vi "Autonomous Independent.vi"   [LabVIEW 2016]
doc: "This VI is called when autonomous begins, and will automatically be terminated when autonomous ends. You can carry out timed or sensor driven robot movement independently without needing to return to the caller."
uses:
  <vilib>/Rock Robotics/Network Tables/NT Read String.vi
  Robot Global Data.vi
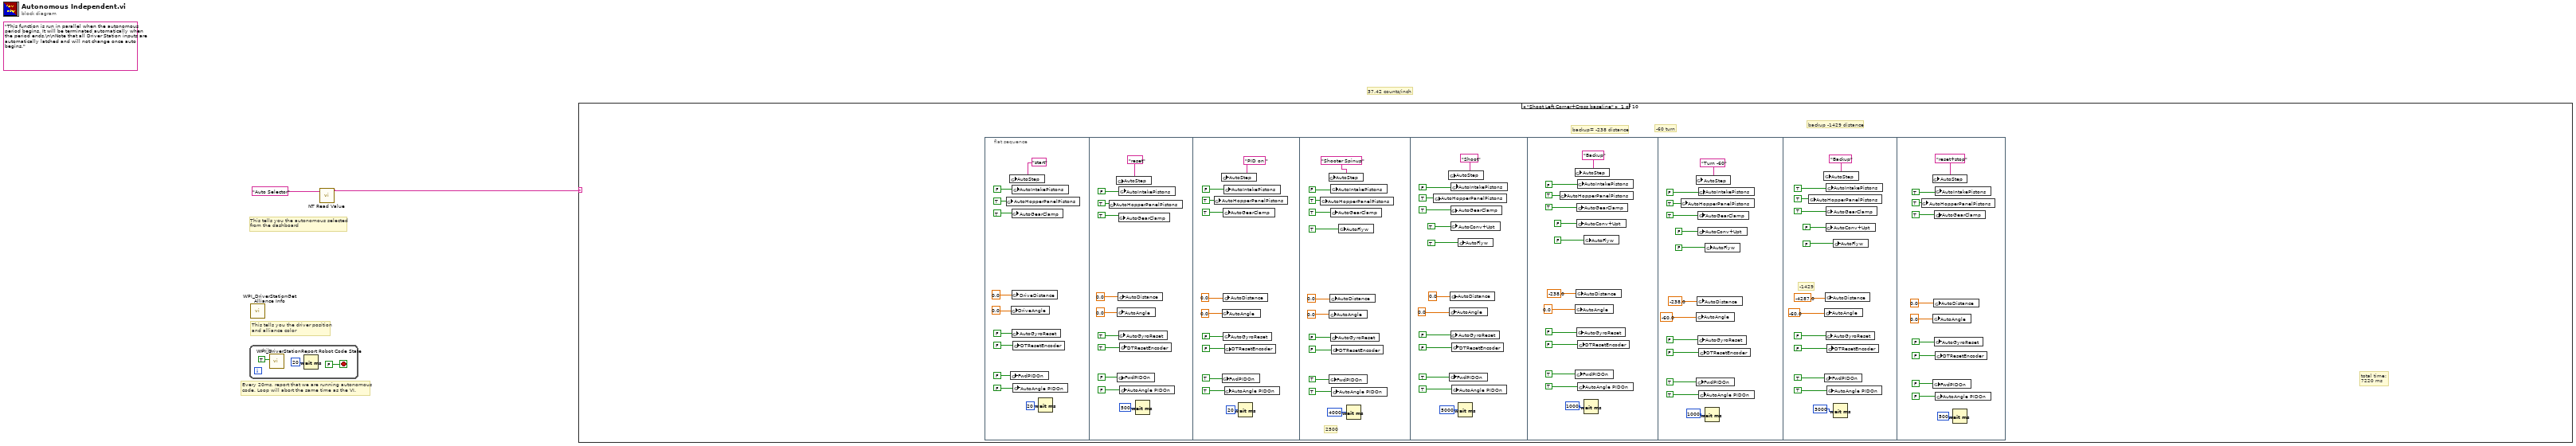
[diagram p0: block diagram]
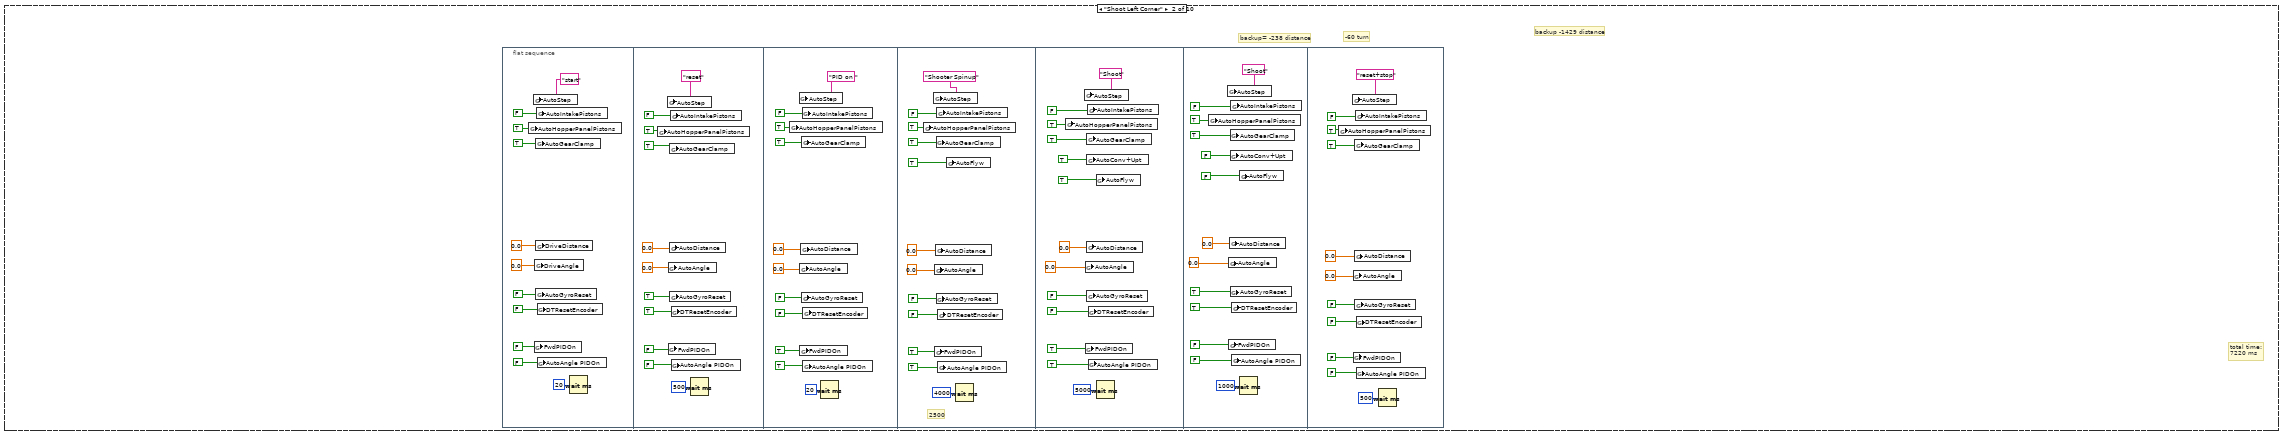
[diagram p2: hidden frame]
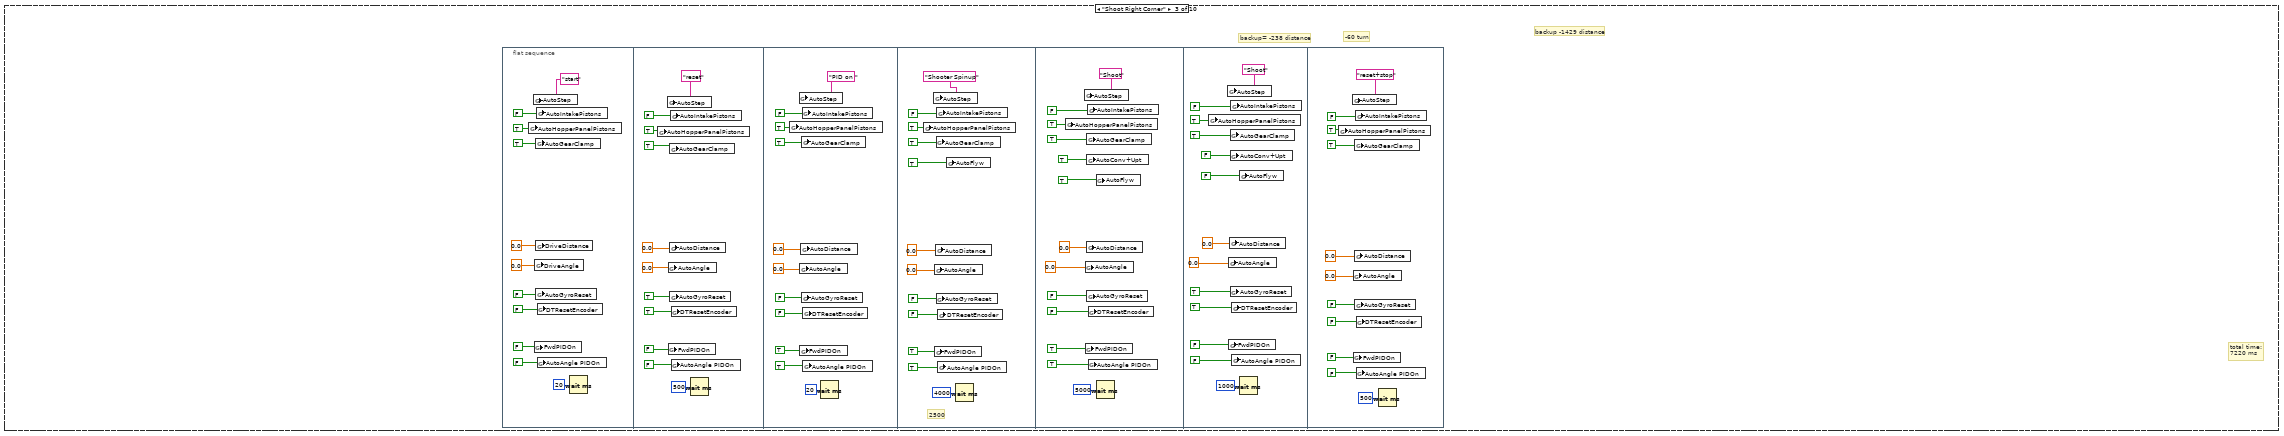
[diagram p3: hidden frame]
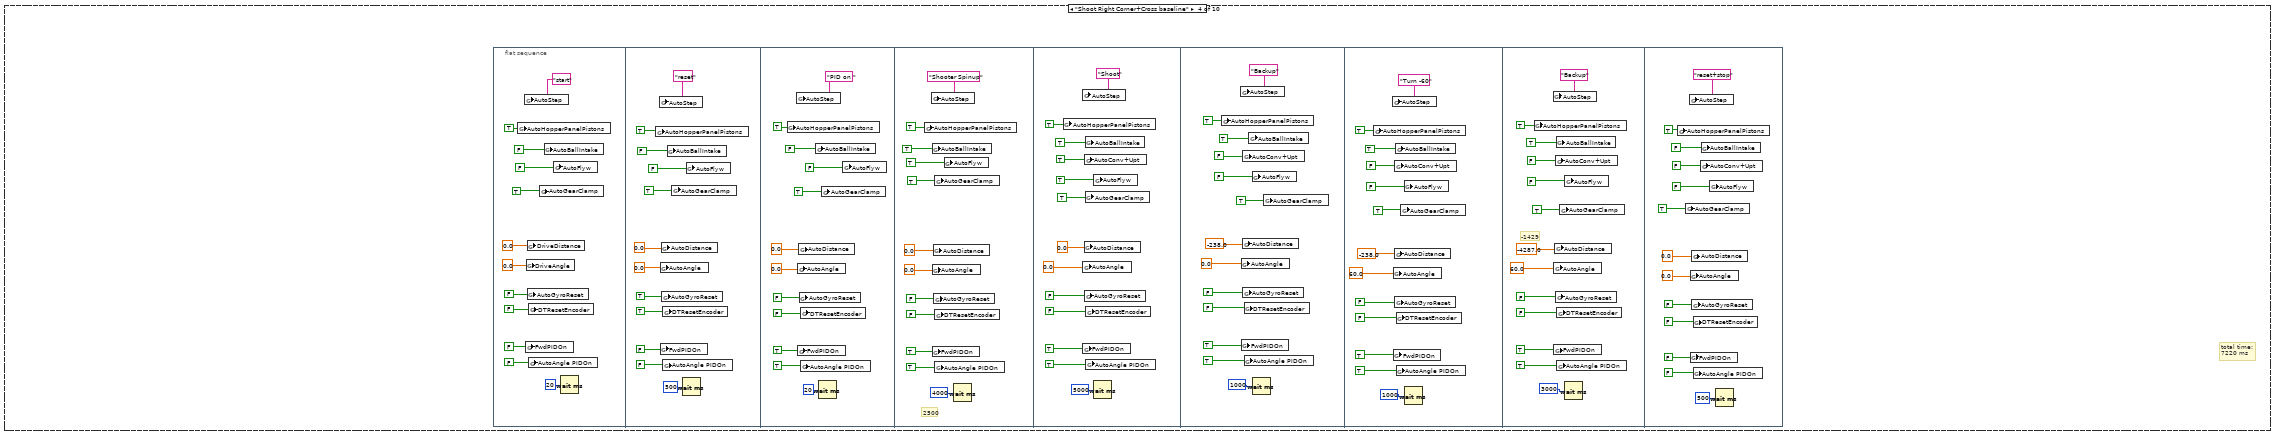
[diagram p4: hidden frame]
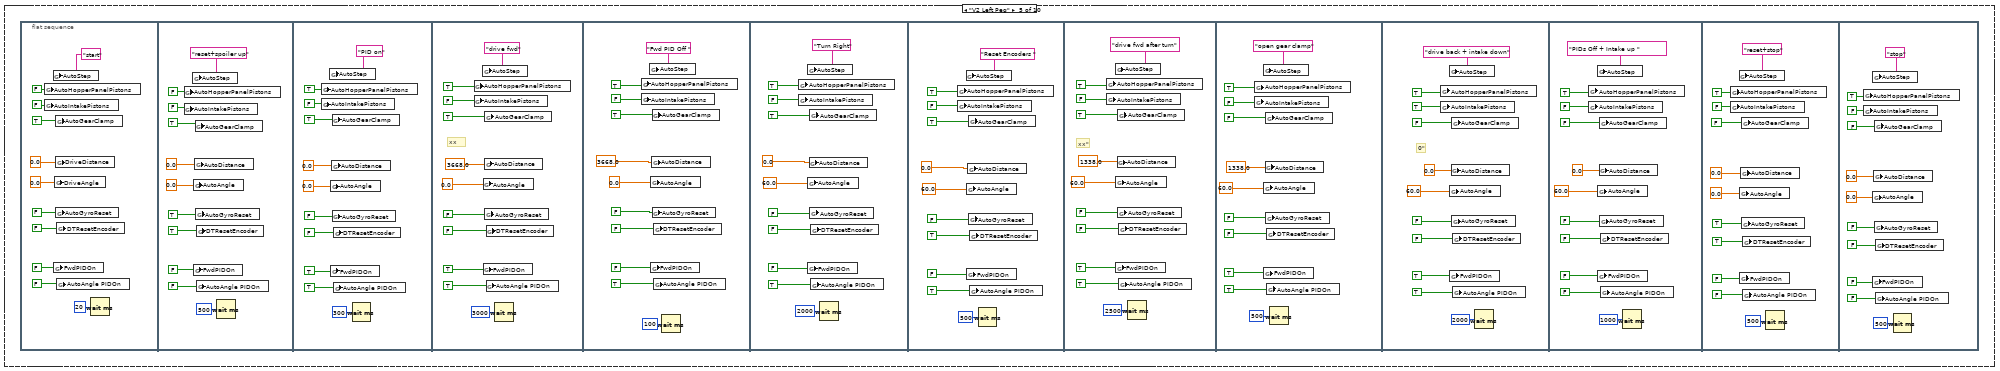
[diagram p5: hidden frame]
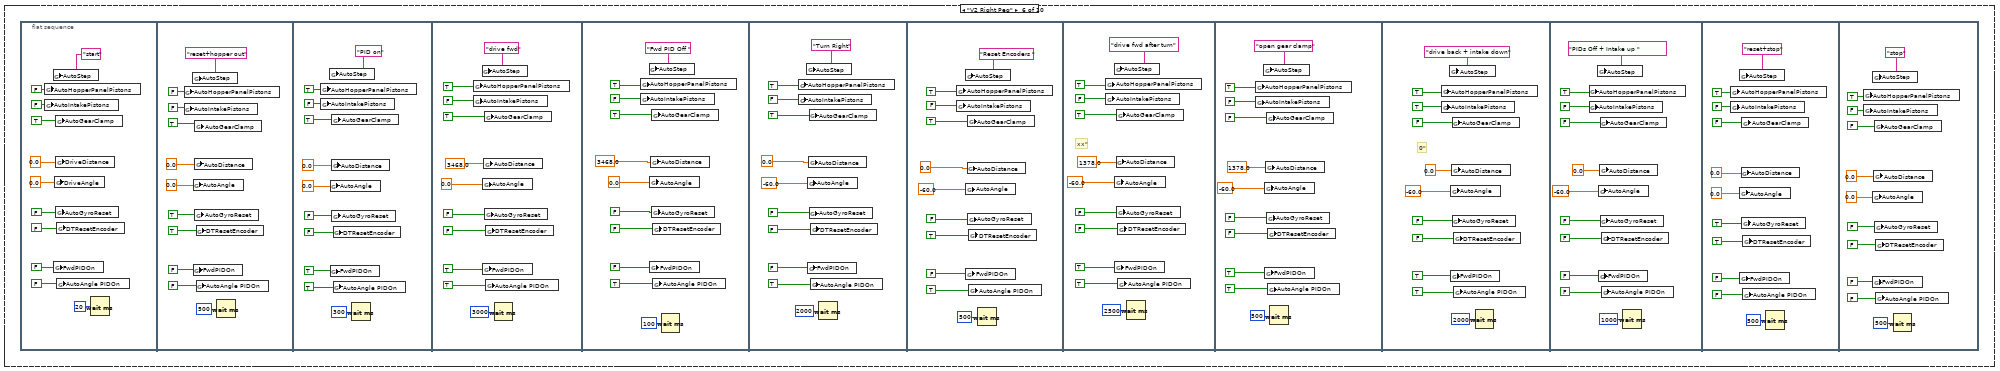
[diagram p6: hidden frame]
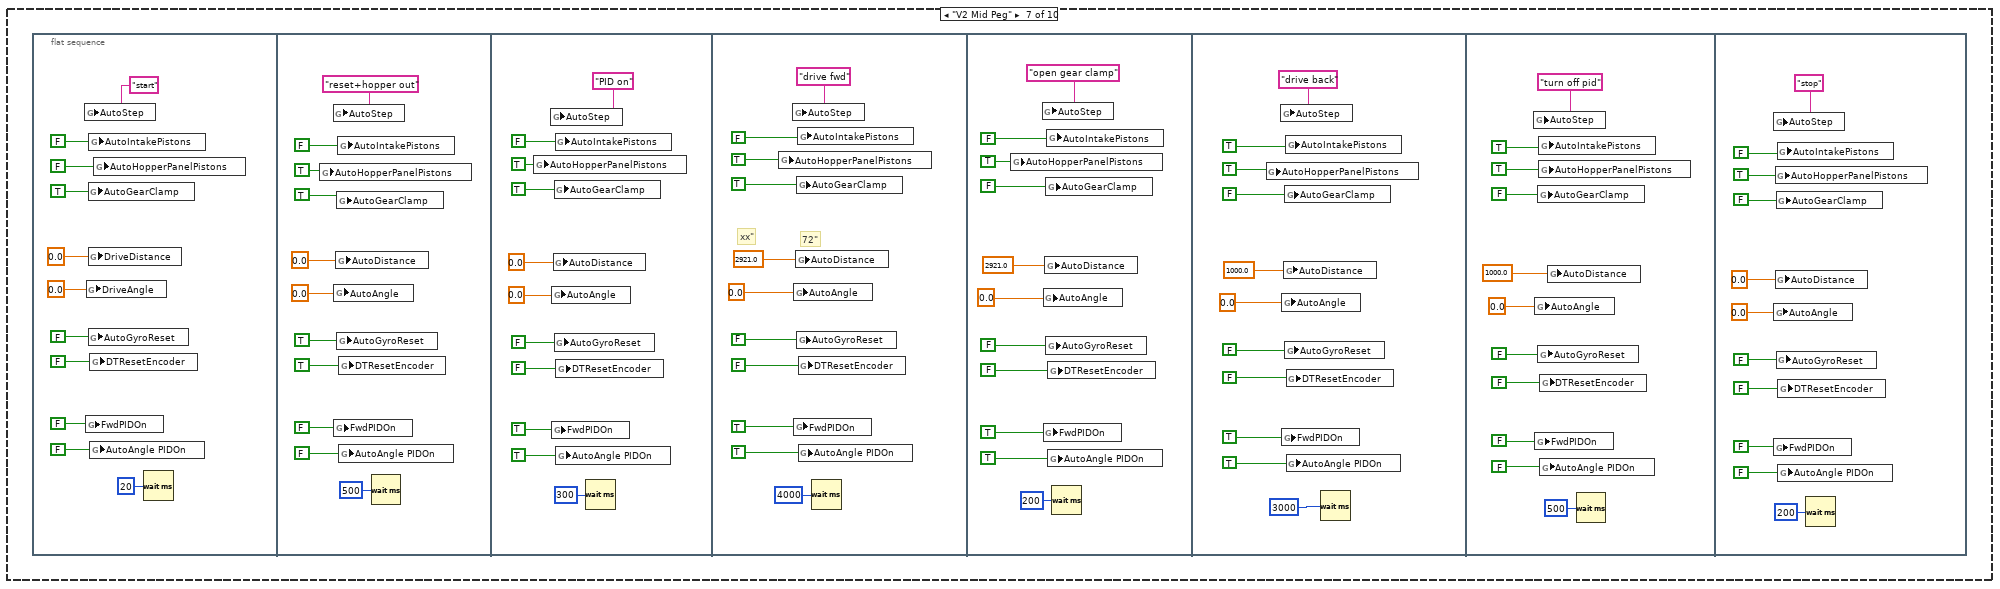
[diagram p7: hidden frame]
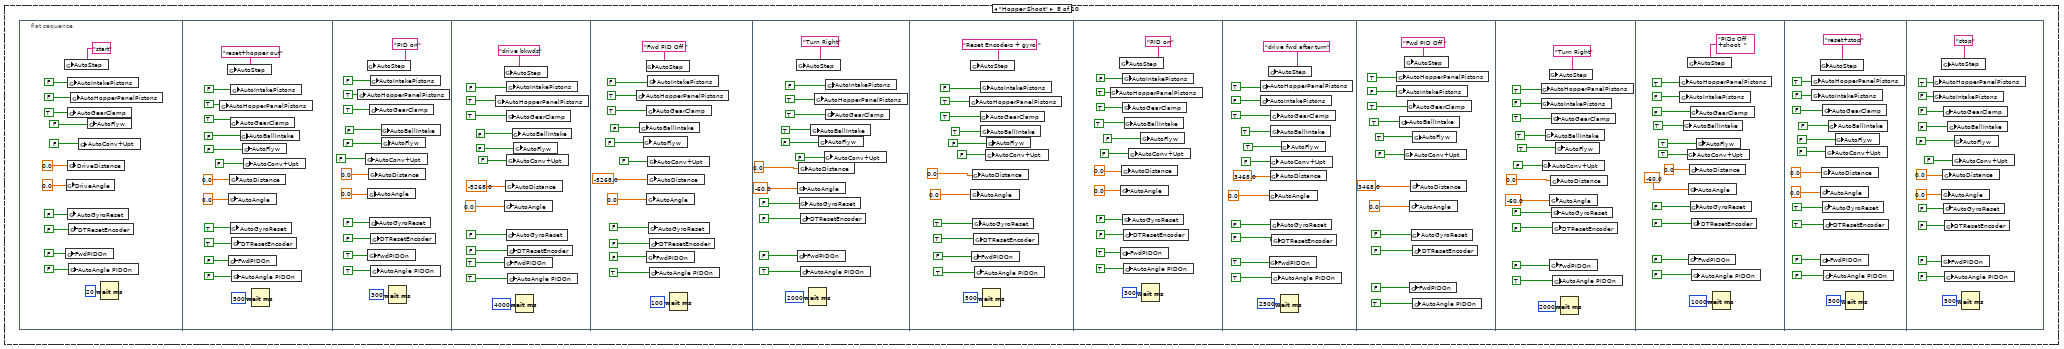
[diagram p8: hidden frame]
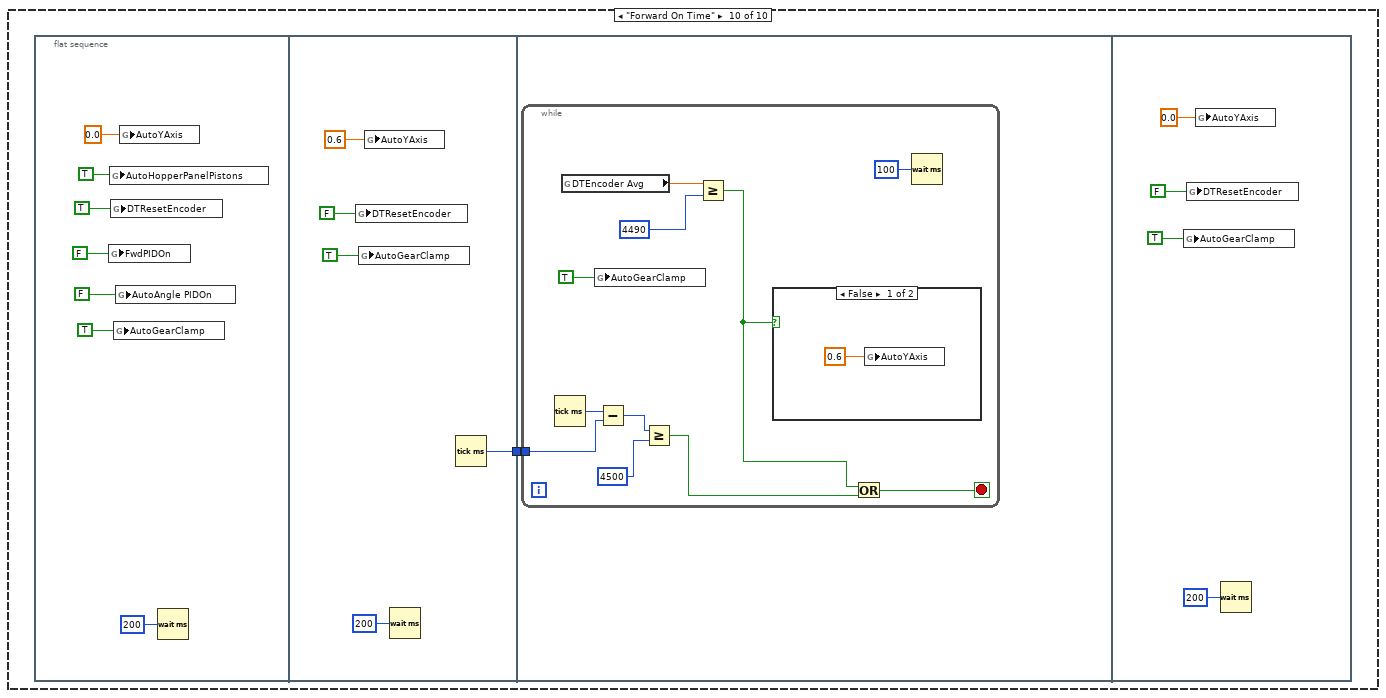
[diagram p10: hidden frame]
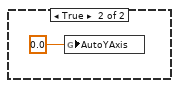
[diagram p11: hidden frame]
diagram:
  (unwired) "This function is run in parallel when the autonomous period begins. It will be terminated automatically when the period ends.\n\nNote that all Driver Station inputs are automatically latched and will not change once auto begins."
  # "37.42 counts/inch"
  # "This tells you the autonomous selected\nfrom the dashboard"
  # "Every 20ms, report that we are running autonomous\ncode. Loop will abort the same time as the VI."
  # "This tells you the driver position\nand alliance color"
  n1 = while {
    stop <- FALSE stop-if-true
    n2 = call <vilib>:"WPI_DriverStationReport Robot Code State.vi"("Autonomous"=TRUE) -> ()  [unwired: 10 in, 1 out]
    n3 = Wait (ms)(milliseconds to wait=u32 20) -> ()  [unwired: 1 out]
  }
  n4 = call <vilib>:"WPI_DriverStationGet Alliance Info.vi"() -> ()  [unwired: 12 out]
  n5 = call-poly <vilib>:"NT Read Value.vi"("Name"="Auto Selector") -> ("String"=w1:string)  [unwired: 9 in, 1 out]
  n6 = case shown="\"Shoot Left Corner+Cross baseline\"" w1 {
    frame "Shoot Left Corner+Cross baseline" {
      # "backup -1429 distance"
      # "-60 turn"
      # "backup= -238 distance"
      # "total time: \n7220 ms"
      n7 = flat-sequence {
        frame #0 {
          n8 = global write "Robot Global Data.vi" "AutoHopperPanelPistons"(TRUE ("GyroReset")) -> ()
          n9 = global write "Robot Global Data.vi" "AutoStep"("start" ("AutoStep")) -> ()
          n10 = global write "Robot Global Data.vi" "FwdPIDOn"(FALSE ("FwdPIDOn")) -> ()
          n11 = global write "Robot Global Data.vi" "DriveAngle"(0.0 ("DriveAngle")) -> ()
          n12 = global write "Robot Global Data.vi" "AutoGearClamp"(TRUE ("DTResetEncoder")) -> ()
          n13 = global write "Robot Global Data.vi" "DriveDistance"(0.0 ("DriveDistance")) -> ()
          n14 = global write "Robot Global Data.vi" "AutoGyroReset"(FALSE ("GyroReset")) -> ()
          n15 = global write "Robot Global Data.vi" "AutoIntakePistons"(FALSE ("GyroReset")) -> ()
          n16 = global write "Robot Global Data.vi" "DTResetEncoder"(FALSE ("DTResetEncoder")) -> ()
          n17 = global write "Robot Global Data.vi" "AutoAngle PIDOn"(FALSE ("AnglePIDOn")) -> ()
          n18 = Wait (ms)(milliseconds to wait=u32 20) -> ()  [unwired: 1 out]
        }
        frame #1 {
          n19 = global write "Robot Global Data.vi" "AutoHopperPanelPistons"(TRUE ("GyroReset")) -> ()
          n20 = global write "Robot Global Data.vi" "AutoStep"("reset" ("AutoStep")) -> ()
          n21 = global write "Robot Global Data.vi" "AutoAngle"(0.0 ("DriveAngle")) -> ()
          n22 = global write "Robot Global Data.vi" "FwdPIDOn"(FALSE ("FwdPIDOn")) -> ()
          n23 = global write "Robot Global Data.vi" "AutoDistance"(0.0 ("DriveDistance")) -> ()
          n24 = global write "Robot Global Data.vi" "AutoGearClamp"(TRUE ("DTResetEncoder")) -> ()
          n25 = global write "Robot Global Data.vi" "AutoGyroReset"(TRUE ("GyroReset")) -> ()
          n26 = global write "Robot Global Data.vi" "AutoIntakePistons"(FALSE ("GyroReset")) -> ()
          n27 = global write "Robot Global Data.vi" "DTResetEncoder"(TRUE ("DTResetEncoder")) -> ()
          n28 = global write "Robot Global Data.vi" "AutoAngle PIDOn"(FALSE ("AnglePIDOn")) -> ()
          n29 = Wait (ms)(milliseconds to wait=u32 500) -> ()  [unwired: 1 out]
        }
        frame #2 {
          n30 = global write "Robot Global Data.vi" "AutoHopperPanelPistons"(TRUE ("GyroReset")) -> ()
          n31 = global write "Robot Global Data.vi" "AutoStep"("PID on " ("AutoStep")) -> ()
          n32 = global write "Robot Global Data.vi" "AutoAngle"(0.0 ("DriveAngle")) -> ()
          n33 = global write "Robot Global Data.vi" "FwdPIDOn"(TRUE ("FwdPIDOn")) -> ()
          n34 = global write "Robot Global Data.vi" "AutoDistance"(0.0 ("DriveDistance")) -> ()
          n35 = global write "Robot Global Data.vi" "AutoGearClamp"(TRUE ("DTResetEncoder")) -> ()
          n36 = global write "Robot Global Data.vi" "AutoGyroReset"(FALSE ("GyroReset")) -> ()
          n37 = global write "Robot Global Data.vi" "AutoIntakePistons"(FALSE ("GyroReset")) -> ()
          n38 = global write "Robot Global Data.vi" "DTResetEncoder"(FALSE ("DTResetEncoder")) -> ()
          n39 = global write "Robot Global Data.vi" "AutoAngle PIDOn"(TRUE ("AnglePIDOn")) -> ()
          n40 = Wait (ms)(milliseconds to wait=u32 20) -> ()  [unwired: 1 out]
        }
        frame #3 {
          # "2500"
          n41 = global write "Robot Global Data.vi" "AutoHopperPanelPistons"(TRUE ("GyroReset")) -> ()
          n42 = global write "Robot Global Data.vi" "AutoStep"("Shooter Spinup" ("AutoStep")) -> ()
          n43 = global write "Robot Global Data.vi" "AutoAngle"(0.0 ("DriveAngle")) -> ()
          n44 = global write "Robot Global Data.vi" "FwdPIDOn"(TRUE ("FwdPIDOn")) -> ()
          n45 = global write "Robot Global Data.vi" "AutoDistance"(0.0 ("DriveDistance")) -> ()
          n46 = global write "Robot Global Data.vi" "AutoGearClamp"(TRUE ("DTResetEncoder")) -> ()
          n47 = global write "Robot Global Data.vi" "AutoGyroReset"(FALSE ("GyroReset")) -> ()
          n48 = global write "Robot Global Data.vi" "AutoIntakePistons"(FALSE ("GyroReset")) -> ()
          n49 = global write "Robot Global Data.vi" "DTResetEncoder"(FALSE ("DTResetEncoder")) -> ()
          n50 = global write "Robot Global Data.vi" "AutoAngle PIDOn"(TRUE ("AnglePIDOn")) -> ()
          n51 = global write "Robot Global Data.vi" "AutoFlyw"(TRUE ("DTResetEncoder")) -> ()
          n52 = Wait (ms)(milliseconds to wait=u32 4000) -> ()  [unwired: 1 out]
        }
        frame #4 {
          n53 = global write "Robot Global Data.vi" "AutoHopperPanelPistons"(TRUE ("GyroReset")) -> ()
          n54 = global write "Robot Global Data.vi" "AutoStep"("Shoot" ("AutoStep")) -> ()
          n55 = global write "Robot Global Data.vi" "AutoAngle"(0.0 ("DriveAngle")) -> ()
          n56 = global write "Robot Global Data.vi" "FwdPIDOn"(TRUE ("FwdPIDOn")) -> ()
          n57 = global write "Robot Global Data.vi" "AutoDistance"(0.0 ("DriveDistance")) -> ()
          n58 = global write "Robot Global Data.vi" "AutoGearClamp"(TRUE ("DTResetEncoder")) -> ()
          n59 = global write "Robot Global Data.vi" "AutoConv+Upt"(TRUE ("DTResetEncoder")) -> ()
          n60 = global write "Robot Global Data.vi" "AutoGyroReset"(FALSE ("GyroReset")) -> ()
          n61 = global write "Robot Global Data.vi" "AutoIntakePistons"(FALSE ("GyroReset")) -> ()
          n62 = global write "Robot Global Data.vi" "DTResetEncoder"(FALSE ("DTResetEncoder")) -> ()
          n63 = global write "Robot Global Data.vi" "AutoAngle PIDOn"(TRUE ("AnglePIDOn")) -> ()
          n64 = global write "Robot Global Data.vi" "AutoFlyw"(TRUE ("DTResetEncoder")) -> ()
          n65 = Wait (ms)(milliseconds to wait=u32 5000) -> ()  [unwired: 1 out]
        }
        frame #5 {
          n66 = global write "Robot Global Data.vi" "AutoHopperPanelPistons"(TRUE ("GyroReset")) -> ()
          n67 = global write "Robot Global Data.vi" "AutoStep"("Backup" ("AutoStep")) -> ()
          n68 = global write "Robot Global Data.vi" "AutoAngle"(0.0 ("DriveAngle")) -> ()
          n69 = global write "Robot Global Data.vi" "FwdPIDOn"(TRUE ("FwdPIDOn")) -> ()
          n70 = global write "Robot Global Data.vi" "AutoDistance"(-238.0 ("DriveDistance")) -> ()
          n71 = global write "Robot Global Data.vi" "AutoGearClamp"(TRUE ("DTResetEncoder")) -> ()
          n72 = global write "Robot Global Data.vi" "AutoConv+Upt"(FALSE ("DTResetEncoder")) -> ()
          n73 = global write "Robot Global Data.vi" "AutoGyroReset"(FALSE ("GyroReset")) -> ()
          n74 = global write "Robot Global Data.vi" "AutoIntakePistons"(FALSE ("GyroReset")) -> ()
          n75 = global write "Robot Global Data.vi" "DTResetEncoder"(FALSE ("DTResetEncoder")) -> ()
          n76 = global write "Robot Global Data.vi" "AutoAngle PIDOn"(TRUE ("AnglePIDOn")) -> ()
          n77 = global write "Robot Global Data.vi" "AutoFlyw"(FALSE ("DTResetEncoder")) -> ()
          n78 = Wait (ms)(milliseconds to wait=u32 1000) -> ()  [unwired: 1 out]
        }
        frame #6 {
          n79 = global write "Robot Global Data.vi" "AutoHopperPanelPistons"(TRUE ("GyroReset")) -> ()
          n80 = global write "Robot Global Data.vi" "AutoStep"("Turn -60" ("AutoStep")) -> ()
          n81 = global write "Robot Global Data.vi" "AutoAngle"(-60.0 ("DriveAngle")) -> ()
          n82 = global write "Robot Global Data.vi" "FwdPIDOn"(TRUE ("FwdPIDOn")) -> ()
          n83 = global write "Robot Global Data.vi" "AutoDistance"(-238.0 ("DriveDistance")) -> ()
          n84 = global write "Robot Global Data.vi" "AutoGearClamp"(TRUE ("DTResetEncoder")) -> ()
          n85 = global write "Robot Global Data.vi" "AutoConv+Upt"(FALSE ("DTResetEncoder")) -> ()
          n86 = global write "Robot Global Data.vi" "AutoGyroReset"(FALSE ("GyroReset")) -> ()
          n87 = global write "Robot Global Data.vi" "AutoIntakePistons"(FALSE ("GyroReset")) -> ()
          n88 = global write "Robot Global Data.vi" "DTResetEncoder"(FALSE ("DTResetEncoder")) -> ()
          n89 = global write "Robot Global Data.vi" "AutoAngle PIDOn"(TRUE ("AnglePIDOn")) -> ()
          n90 = global write "Robot Global Data.vi" "AutoFlyw"(FALSE ("DTResetEncoder")) -> ()
          n91 = Wait (ms)(milliseconds to wait=u32 1000) -> ()  [unwired: 1 out]
        }
        frame #7 {
          # "-1429"
          n92 = global write "Robot Global Data.vi" "AutoHopperPanelPistons"(TRUE ("GyroReset")) -> ()
          n93 = global write "Robot Global Data.vi" "AutoStep"("Backup" ("AutoStep")) -> ()
          n94 = global write "Robot Global Data.vi" "AutoAngle"(-60.0 ("DriveAngle")) -> ()
          n95 = global write "Robot Global Data.vi" "FwdPIDOn"(TRUE ("FwdPIDOn")) -> ()
          n96 = global write "Robot Global Data.vi" "AutoDistance"(-4287.0 ("DriveDistance")) -> ()
          n97 = global write "Robot Global Data.vi" "AutoGearClamp"(TRUE ("DTResetEncoder")) -> ()
          n98 = global write "Robot Global Data.vi" "AutoConv+Upt"(FALSE ("DTResetEncoder")) -> ()
          n99 = global write "Robot Global Data.vi" "AutoGyroReset"(FALSE ("GyroReset")) -> ()
          n100 = global write "Robot Global Data.vi" "AutoIntakePistons"(TRUE ("GyroReset")) -> ()
          n101 = global write "Robot Global Data.vi" "DTResetEncoder"(FALSE ("DTResetEncoder")) -> ()
          n102 = global write "Robot Global Data.vi" "AutoAngle PIDOn"(TRUE ("AnglePIDOn")) -> ()
          n103 = global write "Robot Global Data.vi" "AutoFlyw"(FALSE ("DTResetEncoder")) -> ()
          n104 = Wait (ms)(milliseconds to wait=u32 3000) -> ()  [unwired: 1 out]
        }
        frame #8 {
          n105 = global write "Robot Global Data.vi" "AutoHopperPanelPistons"(TRUE ("GyroReset")) -> ()
          n106 = global write "Robot Global Data.vi" "AutoStep"("reset+stop" ("AutoStep")) -> ()
          n107 = global write "Robot Global Data.vi" "AutoAngle"(0.0 ("DriveAngle")) -> ()
          n108 = global write "Robot Global Data.vi" "FwdPIDOn"(FALSE ("FwdPIDOn")) -> ()
          n109 = global write "Robot Global Data.vi" "AutoDistance"(0.0 ("DriveDistance")) -> ()
          n110 = global write "Robot Global Data.vi" "AutoGearClamp"(TRUE ("DTResetEncoder")) -> ()
          n111 = global write "Robot Global Data.vi" "AutoGyroReset"(FALSE ("GyroReset")) -> ()
          n112 = global write "Robot Global Data.vi" "AutoIntakePistons"(TRUE ("GyroReset")) -> ()
          n113 = global write "Robot Global Data.vi" "DTResetEncoder"(FALSE ("DTResetEncoder")) -> ()
          n114 = global write "Robot Global Data.vi" "AutoAngle PIDOn"(FALSE ("AnglePIDOn")) -> ()
          n115 = Wait (ms)(milliseconds to wait=u32 500) -> ()  [unwired: 1 out]
        }
      }
    }
    frame "Shoot Left Corner" {
      # "backup -1429 distance"
      # "-60 turn"
      # "backup= -238 distance"
      # "total time: \n7220 ms"
      n116 = flat-sequence {
        frame #0 {
          n117 = global write "Robot Global Data.vi" "AutoHopperPanelPistons"(TRUE ("GyroReset")) -> ()
          n118 = global write "Robot Global Data.vi" "AutoStep"("start" ("AutoStep")) -> ()
          n119 = global write "Robot Global Data.vi" "FwdPIDOn"(FALSE ("FwdPIDOn")) -> ()
          n120 = global write "Robot Global Data.vi" "DriveAngle"(0.0 ("DriveAngle")) -> ()
          n121 = global write "Robot Global Data.vi" "AutoGearClamp"(TRUE ("DTResetEncoder")) -> ()
          n122 = global write "Robot Global Data.vi" "DriveDistance"(0.0 ("DriveDistance")) -> ()
          n123 = global write "Robot Global Data.vi" "AutoGyroReset"(FALSE ("GyroReset")) -> ()
          n124 = global write "Robot Global Data.vi" "AutoIntakePistons"(FALSE ("GyroReset")) -> ()
          n125 = global write "Robot Global Data.vi" "DTResetEncoder"(FALSE ("DTResetEncoder")) -> ()
          n126 = global write "Robot Global Data.vi" "AutoAngle PIDOn"(FALSE ("AnglePIDOn")) -> ()
          n127 = Wait (ms)(milliseconds to wait=u32 20) -> ()  [unwired: 1 out]
        }
        frame #1 {
          n128 = global write "Robot Global Data.vi" "AutoHopperPanelPistons"(TRUE ("GyroReset")) -> ()
          n129 = global write "Robot Global Data.vi" "AutoStep"("reset" ("AutoStep")) -> ()
          n130 = global write "Robot Global Data.vi" "AutoAngle"(0.0 ("DriveAngle")) -> ()
          n131 = global write "Robot Global Data.vi" "FwdPIDOn"(FALSE ("FwdPIDOn")) -> ()
          n132 = global write "Robot Global Data.vi" "AutoDistance"(0.0 ("DriveDistance")) -> ()
          n133 = global write "Robot Global Data.vi" "AutoGearClamp"(TRUE ("DTResetEncoder")) -> ()
          n134 = global write "Robot Global Data.vi" "AutoGyroReset"(TRUE ("GyroReset")) -> ()
          n135 = global write "Robot Global Data.vi" "AutoIntakePistons"(FALSE ("GyroReset")) -> ()
          n136 = global write "Robot Global Data.vi" "DTResetEncoder"(TRUE ("DTResetEncoder")) -> ()
          n137 = global write "Robot Global Data.vi" "AutoAngle PIDOn"(FALSE ("AnglePIDOn")) -> ()
          n138 = Wait (ms)(milliseconds to wait=u32 500) -> ()  [unwired: 1 out]
        }
        frame #2 {
          n139 = global write "Robot Global Data.vi" "AutoHopperPanelPistons"(TRUE ("GyroReset")) -> ()
          n140 = global write "Robot Global Data.vi" "AutoStep"("PID on " ("AutoStep")) -> ()
          n141 = global write "Robot Global Data.vi" "AutoAngle"(0.0 ("DriveAngle")) -> ()
          n142 = global write "Robot Global Data.vi" "FwdPIDOn"(TRUE ("FwdPIDOn")) -> ()
          n143 = global write "Robot Global Data.vi" "AutoDistance"(0.0 ("DriveDistance")) -> ()
          n144 = global write "Robot Global Data.vi" "AutoGearClamp"(TRUE ("DTResetEncoder")) -> ()
          n145 = global write "Robot Global Data.vi" "AutoGyroReset"(FALSE ("GyroReset")) -> ()
          n146 = global write "Robot Global Data.vi" "AutoIntakePistons"(FALSE ("GyroReset")) -> ()
          n147 = global write "Robot Global Data.vi" "DTResetEncoder"(FALSE ("DTResetEncoder")) -> ()
          n148 = global write "Robot Global Data.vi" "AutoAngle PIDOn"(TRUE ("AnglePIDOn")) -> ()
          n149 = Wait (ms)(milliseconds to wait=u32 20) -> ()  [unwired: 1 out]
        }
        frame #3 {
          # "2500"
          n150 = global write "Robot Global Data.vi" "AutoHopperPanelPistons"(TRUE ("GyroReset")) -> ()
          n151 = global write "Robot Global Data.vi" "AutoStep"("Shooter Spinup" ("AutoStep")) -> ()
          n152 = global write "Robot Global Data.vi" "AutoAngle"(0.0 ("DriveAngle")) -> ()
          n153 = global write "Robot Global Data.vi" "FwdPIDOn"(TRUE ("FwdPIDOn")) -> ()
          n154 = global write "Robot Global Data.vi" "AutoDistance"(0.0 ("DriveDistance")) -> ()
          n155 = global write "Robot Global Data.vi" "AutoGearClamp"(TRUE ("DTResetEncoder")) -> ()
          n156 = global write "Robot Global Data.vi" "AutoGyroReset"(FALSE ("GyroReset")) -> ()
          n157 = global write "Robot Global Data.vi" "AutoIntakePistons"(FALSE ("GyroReset")) -> ()
          n158 = global write "Robot Global Data.vi" "DTResetEncoder"(FALSE ("DTResetEncoder")) -> ()
          n159 = global write "Robot Global Data.vi" "AutoAngle PIDOn"(TRUE ("AnglePIDOn")) -> ()
          n160 = global write "Robot Global Data.vi" "AutoFlyw"(TRUE ("DTResetEncoder")) -> ()
          n161 = Wait (ms)(milliseconds to wait=u32 4000) -> ()  [unwired: 1 out]
        }
        frame #4 {
          n162 = global write "Robot Global Data.vi" "AutoHopperPanelPistons"(TRUE ("GyroReset")) -> ()
          n163 = global write "Robot Global Data.vi" "AutoStep"("Shoot" ("AutoStep")) -> ()
          n164 = global write "Robot Global Data.vi" "AutoAngle"(0.0 ("DriveAngle")) -> ()
          n165 = global write "Robot Global Data.vi" "FwdPIDOn"(TRUE ("FwdPIDOn")) -> ()
          n166 = global write "Robot Global Data.vi" "AutoDistance"(0.0 ("DriveDistance")) -> ()
          n167 = global write "Robot Global Data.vi" "AutoGearClamp"(TRUE ("DTResetEncoder")) -> ()
          n168 = global write "Robot Global Data.vi" "AutoConv+Upt"(TRUE ("DTResetEncoder")) -> ()
          n169 = global write "Robot Global Data.vi" "AutoGyroReset"(FALSE ("GyroReset")) -> ()
          n170 = global write "Robot Global Data.vi" "AutoIntakePistons"(FALSE ("GyroReset")) -> ()
          n171 = global write "Robot Global Data.vi" "DTResetEncoder"(FALSE ("DTResetEncoder")) -> ()
          n172 = global write "Robot Global Data.vi" "AutoAngle PIDOn"(TRUE ("AnglePIDOn")) -> ()
          n173 = global write "Robot Global Data.vi" "AutoFlyw"(TRUE ("DTResetEncoder")) -> ()
          n174 = Wait (ms)(milliseconds to wait=u32 5000) -> ()  [unwired: 1 out]
        }
        frame #5 {
          n175 = global write "Robot Global Data.vi" "AutoHopperPanelPistons"(TRUE ("GyroReset")) -> ()
          n176 = global write "Robot Global Data.vi" "AutoStep"("Shoot" ("AutoStep")) -> ()
          n177 = global write "Robot Global Data.vi" "AutoAngle"(0.0 ("DriveAngle")) -> ()
          n178 = global write "Robot Global Data.vi" "FwdPIDOn"(FALSE ("FwdPIDOn")) -> ()
          n179 = global write "Robot Global Data.vi" "AutoDistance"(0.0 ("DriveDistance")) -> ()
          n180 = global write "Robot Global Data.vi" "AutoGearClamp"(TRUE ("DTResetEncoder")) -> ()
          n181 = global write "Robot Global Data.vi" "AutoConv+Upt"(FALSE ("DTResetEncoder")) -> ()
          n182 = global write "Robot Global Data.vi" "AutoGyroReset"(TRUE ("GyroReset")) -> ()
          n183 = global write "Robot Global Data.vi" "AutoIntakePistons"(FALSE ("GyroReset")) -> ()
          n184 = global write "Robot Global Data.vi" "DTResetEncoder"(TRUE ("DTResetEncoder")) -> ()
          n185 = global write "Robot Global Data.vi" "AutoAngle PIDOn"(FALSE ("AnglePIDOn")) -> ()
          n186 = global write "Robot Global Data.vi" "AutoFlyw"(FALSE ("DTResetEncoder")) -> ()
          n187 = Wait (ms)(milliseconds to wait=u32 1000) -> ()  [unwired: 1 out]
        }
        frame #6 {
          n188 = global write "Robot Global Data.vi" "AutoHopperPanelPistons"(TRUE ("GyroReset")) -> ()
          n189 = global write "Robot Global Data.vi" "AutoStep"("reset+stop" ("AutoStep")) -> ()
          n190 = global write "Robot Global Data.vi" "AutoAngle"(0.0 ("DriveAngle")) -> ()
          n191 = global write "Robot Global Data.vi" "FwdPIDOn"(FALSE ("FwdPIDOn")) -> ()
          n192 = global write "Robot Global Data.vi" "AutoDistance"(0.0 ("DriveDistance")) -> ()
          n193 = global write "Robot Global Data.vi" "AutoGearClamp"(TRUE ("DTResetEncoder")) -> ()
          n194 = global write "Robot Global Data.vi" "AutoGyroReset"(FALSE ("GyroReset")) -> ()
          n195 = global write "Robot Global Data.vi" "AutoIntakePistons"(FALSE ("GyroReset")) -> ()
          n196 = global write "Robot Global Data.vi" "DTResetEncoder"(FALSE ("DTResetEncoder")) -> ()
          n197 = global write "Robot Global Data.vi" "AutoAngle PIDOn"(FALSE ("AnglePIDOn")) -> ()
          n198 = Wait (ms)(milliseconds to wait=u32 500) -> ()  [unwired: 1 out]
        }
      }
    }
    frame "Shoot Right Corner" {
      # "backup -1429 distance"
      # "-60 turn"
      # "backup= -238 distance"
      # "total time: \n7220 ms"
      n199 = flat-sequence {
        frame #0 {
          n200 = global write "Robot Global Data.vi" "AutoHopperPanelPistons"(TRUE ("GyroReset")) -> ()
          n201 = global write "Robot Global Data.vi" "AutoStep"("start" ("AutoStep")) -> ()
          n202 = global write "Robot Global Data.vi" "FwdPIDOn"(FALSE ("FwdPIDOn")) -> ()
          n203 = global write "Robot Global Data.vi" "DriveAngle"(0.0 ("DriveAngle")) -> ()
          n204 = global write "Robot Global Data.vi" "AutoGearClamp"(TRUE ("DTResetEncoder")) -> ()
          n205 = global write "Robot Global Data.vi" "DriveDistance"(0.0 ("DriveDistance")) -> ()
          n206 = global write "Robot Global Data.vi" "AutoGyroReset"(FALSE ("GyroReset")) -> ()
          n207 = global write "Robot Global Data.vi" "AutoIntakePistons"(FALSE ("GyroReset")) -> ()
          n208 = global write "Robot Global Data.vi" "DTResetEncoder"(FALSE ("DTResetEncoder")) -> ()
          n209 = global write "Robot Global Data.vi" "AutoAngle PIDOn"(FALSE ("AnglePIDOn")) -> ()
          n210 = Wait (ms)(milliseconds to wait=u32 20) -> ()  [unwired: 1 out]
        }
        frame #1 {
          n211 = global write "Robot Global Data.vi" "AutoHopperPanelPistons"(TRUE ("GyroReset")) -> ()
          n212 = global write "Robot Global Data.vi" "AutoStep"("reset" ("AutoStep")) -> ()
          n213 = global write "Robot Global Data.vi" "AutoAngle"(0.0 ("DriveAngle")) -> ()
          n214 = global write "Robot Global Data.vi" "FwdPIDOn"(FALSE ("FwdPIDOn")) -> ()
          n215 = global write "Robot Global Data.vi" "AutoDistance"(0.0 ("DriveDistance")) -> ()
          n216 = global write "Robot Global Data.vi" "AutoGearClamp"(TRUE ("DTResetEncoder")) -> ()
          n217 = global write "Robot Global Data.vi" "AutoGyroReset"(TRUE ("GyroReset")) -> ()
          n218 = global write "Robot Global Data.vi" "AutoIntakePistons"(FALSE ("GyroReset")) -> ()
          n219 = global write "Robot Global Data.vi" "DTResetEncoder"(TRUE ("DTResetEncoder")) -> ()
          n220 = global write "Robot Global Data.vi" "AutoAngle PIDOn"(FALSE ("AnglePIDOn")) -> ()
          n221 = Wait (ms)(milliseconds to wait=u32 500) -> ()  [unwired: 1 out]
        }
        frame #2 {
          n222 = global write "Robot Global Data.vi" "AutoHopperPanelPistons"(TRUE ("GyroReset")) -> ()
          n223 = global write "Robot Global Data.vi" "AutoStep"("PID on " ("AutoStep")) -> ()
          n224 = global write "Robot Global Data.vi" "AutoAngle"(0.0 ("DriveAngle")) -> ()
          n225 = global write "Robot Global Data.vi" "FwdPIDOn"(TRUE ("FwdPIDOn")) -> ()
          n226 = global write "Robot Global Data.vi" "AutoDistance"(0.0 ("DriveDistance")) -> ()
          n227 = global write "Robot Global Data.vi" "AutoGearClamp"(TRUE ("DTResetEncoder")) -> ()
          n228 = global write "Robot Global Data.vi" "AutoGyroReset"(FALSE ("GyroReset")) -> ()
          n229 = global write "Robot Global Data.vi" "AutoIntakePistons"(FALSE ("GyroReset")) -> ()
          n230 = global write "Robot Global Data.vi" "DTResetEncoder"(FALSE ("DTResetEncoder")) -> ()
          n231 = global write "Robot Global Data.vi" "AutoAngle PIDOn"(TRUE ("AnglePIDOn")) -> ()
          n232 = Wait (ms)(milliseconds to wait=u32 20) -> ()  [unwired: 1 out]
        }
        frame #3 {
          # "2500"
          n233 = global write "Robot Global Data.vi" "AutoHopperPanelPistons"(TRUE ("GyroReset")) -> ()
          n234 = global write "Robot Global Data.vi" "AutoStep"("Shooter Spinup" ("AutoStep")) -> ()
          n235 = global write "Robot Global Data.vi" "AutoAngle"(0.0 ("DriveAngle")) -> ()
          n236 = global write "Robot Global Data.vi" "FwdPIDOn"(TRUE ("FwdPIDOn")) -> ()
          n237 = global write "Robot Global Data.vi" "AutoDistance"(0.0 ("DriveDistance")) -> ()
          n238 = global write "Robot Global Data.vi" "AutoGearClamp"(TRUE ("DTResetEncoder")) -> ()
          n239 = global write "Robot Global Data.vi" "AutoGyroReset"(FALSE ("GyroReset")) -> ()
          n240 = global write "Robot Global Data.vi" "AutoIntakePistons"(FALSE ("GyroReset")) -> ()
          n241 = global write "Robot Global Data.vi" "DTResetEncoder"(FALSE ("DTResetEncoder")) -> ()
          n242 = global write "Robot Global Data.vi" "AutoAngle PIDOn"(TRUE ("AnglePIDOn")) -> ()
          n243 = global write "Robot Global Data.vi" "AutoFlyw"(TRUE ("DTResetEncoder")) -> ()
          n244 = Wait (ms)(milliseconds to wait=u32 4000) -> ()  [unwired: 1 out]
        }
        frame #4 {
          n245 = global write "Robot Global Data.vi" "AutoHopperPanelPistons"(TRUE ("GyroReset")) -> ()
          n246 = global write "Robot Global Data.vi" "AutoStep"("Shoot" ("AutoStep")) -> ()
          n247 = global write "Robot Global Data.vi" "AutoAngle"(0.0 ("DriveAngle")) -> ()
          n248 = global write "Robot Global Data.vi" "FwdPIDOn"(TRUE ("FwdPIDOn")) -> ()
          n249 = global write "Robot Global Data.vi" "AutoDistance"(0.0 ("DriveDistance")) -> ()
          n250 = global write "Robot Global Data.vi" "AutoGearClamp"(TRUE ("DTResetEncoder")) -> ()
          n251 = global write "Robot Global Data.vi" "AutoConv+Upt"(TRUE ("DTResetEncoder")) -> ()
          n252 = global write "Robot Global Data.vi" "AutoGyroReset"(FALSE ("GyroReset")) -> ()
          n253 = global write "Robot Global Data.vi" "AutoIntakePistons"(FALSE ("GyroReset")) -> ()
          n254 = global write "Robot Global Data.vi" "DTResetEncoder"(FALSE ("DTResetEncoder")) -> ()
          n255 = global write "Robot Global Data.vi" "AutoAngle PIDOn"(TRUE ("AnglePIDOn")) -> ()
          n256 = global write "Robot Global Data.vi" "AutoFlyw"(TRUE ("DTResetEncoder")) -> ()
          n257 = Wait (ms)(milliseconds to wait=u32 5000) -> ()  [unwired: 1 out]
        }
        frame #5 {
          n258 = global write "Robot Global Data.vi" "AutoHopperPanelPistons"(TRUE ("GyroReset")) -> ()
          n259 = global write "Robot Global Data.vi" "AutoStep"("Shoot" ("AutoStep")) -> ()
          n260 = global write "Robot Global Data.vi" "AutoAngle"(0.0 ("DriveAngle")) -> ()
          n261 = global write "Robot Global Data.vi" "FwdPIDOn"(FALSE ("FwdPIDOn")) -> ()
          n262 = global write "Robot Global Data.vi" "AutoDistance"(0.0 ("DriveDistance")) -> ()
          n263 = global write "Robot Global Data.vi" "AutoGearClamp"(TRUE ("DTResetEncoder")) -> ()
          n264 = global write "Robot Global Data.vi" "AutoConv+Upt"(FALSE ("DTResetEncoder")) -> ()
          n265 = global write "Robot Global Data.vi" "AutoGyroReset"(TRUE ("GyroReset")) -> ()
          n266 = global write "Robot Global Data.vi" "AutoIntakePistons"(FALSE ("GyroReset")) -> ()
          n267 = global write "Robot Global Data.vi" "DTResetEncoder"(TRUE ("DTResetEncoder")) -> ()
          n268 = global write "Robot Global Data.vi" "AutoAngle PIDOn"(FALSE ("AnglePIDOn")) -> ()
          n269 = global write "Robot Global Data.vi" "AutoFlyw"(FALSE ("DTResetEncoder")) -> ()
          n270 = Wait (ms)(milliseconds to wait=u32 1000) -> ()  [unwired: 1 out]
        }
        frame #6 {
          n271 = global write "Robot Global Data.vi" "AutoHopperPanelPistons"(TRUE ("GyroReset")) -> ()
          n272 = global write "Robot Global Data.vi" "AutoStep"("reset+stop" ("AutoStep")) -> ()
          n273 = global write "Robot Global Data.vi" "AutoAngle"(0.0 ("DriveAngle")) -> ()
          n274 = global write "Robot Global Data.vi" "FwdPIDOn"(FALSE ("FwdPIDOn")) -> ()
          n275 = global write "Robot Global Data.vi" "AutoDistance"(0.0 ("DriveDistance")) -> ()
          n276 = global write "Robot Global Data.vi" "AutoGearClamp"(TRUE ("DTResetEncoder")) -> ()
          n277 = global write "Robot Global Data.vi" "AutoGyroReset"(FALSE ("GyroReset")) -> ()
          n278 = global write "Robot Global Data.vi" "AutoIntakePistons"(FALSE ("GyroReset")) -> ()
          n279 = global write "Robot Global Data.vi" "DTResetEncoder"(FALSE ("DTResetEncoder")) -> ()
          n280 = global write "Robot Global Data.vi" "AutoAngle PIDOn"(FALSE ("AnglePIDOn")) -> ()
          n281 = Wait (ms)(milliseconds to wait=u32 500) -> ()  [unwired: 1 out]
        }
      }
    }
    frame "Shoot Right Corner+Cross baseline" {
      # "total time: \n7220 ms"
      n282 = flat-sequence {
        frame #0 {
          n283 = global write "Robot Global Data.vi" "AutoHopperPanelPistons"(TRUE ("GyroReset")) -> ()
          n284 = global write "Robot Global Data.vi" "AutoStep"("start" ("AutoStep")) -> ()
          n285 = global write "Robot Global Data.vi" "FwdPIDOn"(FALSE ("FwdPIDOn")) -> ()
          n286 = global write "Robot Global Data.vi" "DriveAngle"(0.0 ("DriveAngle")) -> ()
          n287 = global write "Robot Global Data.vi" "DriveDistance"(0.0 ("DriveDistance")) -> ()
          n288 = global write "Robot Global Data.vi" "AutoGyroReset"(FALSE ("GyroReset")) -> ()
          n289 = global write "Robot Global Data.vi" "DTResetEncoder"(FALSE ("DTResetEncoder")) -> ()
          n290 = global write "Robot Global Data.vi" "AutoAngle PIDOn"(FALSE ("AnglePIDOn")) -> ()
          n291 = global write "Robot Global Data.vi" "AutoGearClamp"(TRUE ("DTResetEncoder")) -> ()
          n292 = global write "Robot Global Data.vi" "AutoBallIntake"(FALSE ("DTResetEncoder")) -> ()
          n293 = global write "Robot Global Data.vi" "AutoFlyw"(FALSE ("DTResetEncoder")) -> ()
          n294 = Wait (ms)(milliseconds to wait=u32 20) -> ()  [unwired: 1 out]
        }
        frame #1 {
          n295 = global write "Robot Global Data.vi" "AutoHopperPanelPistons"(TRUE ("GyroReset")) -> ()
          n296 = global write "Robot Global Data.vi" "AutoStep"("reset" ("AutoStep")) -> ()
          n297 = global write "Robot Global Data.vi" "AutoAngle"(0.0 ("DriveAngle")) -> ()
          n298 = global write "Robot Global Data.vi" "FwdPIDOn"(FALSE ("FwdPIDOn")) -> ()
          n299 = global write "Robot Global Data.vi" "AutoDistance"(0.0 ("DriveDistance")) -> ()
          n300 = global write "Robot Global Data.vi" "AutoGyroReset"(TRUE ("GyroReset")) -> ()
          n301 = global write "Robot Global Data.vi" "DTResetEncoder"(TRUE ("DTResetEncoder")) -> ()
          n302 = global write "Robot Global Data.vi" "AutoAngle PIDOn"(FALSE ("AnglePIDOn")) -> ()
          n303 = global write "Robot Global Data.vi" "AutoBallIntake"(FALSE ("DTResetEncoder")) -> ()
          n304 = global write "Robot Global Data.vi" "AutoGearClamp"(TRUE ("DTResetEncoder")) -> ()
          n305 = Wait (ms)(milliseconds to wait=u32 500) -> ()  [unwired: 1 out]
          n306 = global write "Robot Global Data.vi" "AutoFlyw"(FALSE ("DTResetEncoder")) -> ()
        }
        frame #2 {
          n307 = global write "Robot Global Data.vi" "AutoHopperPanelPistons"(TRUE ("GyroReset")) -> ()
          n308 = global write "Robot Global Data.vi" "AutoStep"("PID on " ("AutoStep")) -> ()
          n309 = global write "Robot Global Data.vi" "AutoAngle"(0.0 ("DriveAngle")) -> ()
          n310 = global write "Robot Global Data.vi" "FwdPIDOn"(TRUE ("FwdPIDOn")) -> ()
          n311 = global write "Robot Global Data.vi" "AutoDistance"(0.0 ("DriveDistance")) -> ()
          n312 = global write "Robot Global Data.vi" "AutoGyroReset"(FALSE ("GyroReset")) -> ()
          n313 = global write "Robot Global Data.vi" "DTResetEncoder"(FALSE ("DTResetEncoder")) -> ()
          n314 = global write "Robot Global Data.vi" "AutoAngle PIDOn"(TRUE ("AnglePIDOn")) -> ()
          n315 = global write "Robot Global Data.vi" "AutoBallIntake"(FALSE ("DTResetEncoder")) -> ()
          n316 = Wait (ms)(milliseconds to wait=u32 20) -> ()  [unwired: 1 out]
          n317 = global write "Robot Global Data.vi" "AutoGearClamp"(TRUE ("DTResetEncoder")) -> ()
          n318 = global write "Robot Global Data.vi" "AutoFlyw"(FALSE ("DTResetEncoder")) -> ()
        }
        frame #3 {
          # "2500"
          n319 = global write "Robot Global Data.vi" "AutoHopperPanelPistons"(TRUE ("GyroReset")) -> ()
          n320 = global write "Robot Global Data.vi" "AutoStep"("Shooter Spinup" ("AutoStep")) -> ()
          n321 = global write "Robot Global Data.vi" "AutoBallIntake"(TRUE ("DTResetEncoder")) -> ()
          n322 = global write "Robot Global Data.vi" "AutoAngle"(0.0 ("DriveAngle")) -> ()
          n323 = global write "Robot Global Data.vi" "FwdPIDOn"(TRUE ("FwdPIDOn")) -> ()
          n324 = global write "Robot Global Data.vi" "AutoDistance"(0.0 ("DriveDistance")) -> ()
          n325 = global write "Robot Global Data.vi" "AutoGyroReset"(FALSE ("GyroReset")) -> ()
          n326 = global write "Robot Global Data.vi" "AutoGearClamp"(TRUE ("DTResetEncoder")) -> ()
          n327 = global write "Robot Global Data.vi" "DTResetEncoder"(FALSE ("DTResetEncoder")) -> ()
          n328 = global write "Robot Global Data.vi" "AutoAngle PIDOn"(TRUE ("AnglePIDOn")) -> ()
          n329 = global write "Robot Global Data.vi" "AutoFlyw"(TRUE ("DTResetEncoder")) -> ()
          n330 = Wait (ms)(milliseconds to wait=u32 4000) -> ()  [unwired: 1 out]
        }
        frame #4 {
          n331 = global write "Robot Global Data.vi" "AutoHopperPanelPistons"(TRUE ("GyroReset")) -> ()
          n332 = global write "Robot Global Data.vi" "AutoStep"("Shoot" ("AutoStep")) -> ()
          n333 = global write "Robot Global Data.vi" "AutoAngle"(0.0 ("DriveAngle")) -> ()
          n334 = global write "Robot Global Data.vi" "FwdPIDOn"(TRUE ("FwdPIDOn")) -> ()
          n335 = global write "Robot Global Data.vi" "AutoDistance"(0.0 ("DriveDistance")) -> ()
          n336 = global write "Robot Global Data.vi" "AutoConv+Upt"(TRUE ("DTResetEncoder")) -> ()
          n337 = global write "Robot Global Data.vi" "AutoGyroReset"(FALSE ("GyroReset")) -> ()
          n338 = global write "Robot Global Data.vi" "AutoBallIntake"(TRUE ("DTResetEncoder")) -> ()
          n339 = global write "Robot Global Data.vi" "AutoGearClamp"(TRUE ("DTResetEncoder")) -> ()
          n340 = global write "Robot Global Data.vi" "DTResetEncoder"(FALSE ("DTResetEncoder")) -> ()
          n341 = global write "Robot Global Data.vi" "AutoAngle PIDOn"(TRUE ("AnglePIDOn")) -> ()
          n342 = global write "Robot Global Data.vi" "AutoFlyw"(TRUE ("DTResetEncoder")) -> ()
          n343 = Wait (ms)(milliseconds to wait=u32 5000) -> ()  [unwired: 1 out]
        }
        frame #5 {
          n344 = global write "Robot Global Data.vi" "AutoHopperPanelPistons"(TRUE ("GyroReset")) -> ()
          n345 = global write "Robot Global Data.vi" "AutoStep"("Backup" ("AutoStep")) -> ()
          n346 = global write "Robot Global Data.vi" "AutoAngle"(0.0 ("DriveAngle")) -> ()
          n347 = global write "Robot Global Data.vi" "FwdPIDOn"(TRUE ("FwdPIDOn")) -> ()
          n348 = global write "Robot Global Data.vi" "AutoDistance"(-238.0 ("DriveDistance")) -> ()
          n349 = global write "Robot Global Data.vi" "AutoConv+Upt"(FALSE ("DTResetEncoder")) -> ()
          n350 = global write "Robot Global Data.vi" "AutoGyroReset"(FALSE ("GyroReset")) -> ()
          n351 = global write "Robot Global Data.vi" "DTResetEncoder"(FALSE ("DTResetEncoder")) -> ()
          n352 = global write "Robot Global Data.vi" "AutoAngle PIDOn"(TRUE ("AnglePIDOn")) -> ()
          n353 = global write "Robot Global Data.vi" "AutoBallIntake"(TRUE ("DTResetEncoder")) -> ()
          n354 = global write "Robot Global Data.vi" "AutoFlyw"(FALSE ("DTResetEncoder")) -> ()
          n355 = Wait (ms)(milliseconds to wait=u32 1000) -> ()  [unwired: 1 out]
          n356 = global write "Robot Global Data.vi" "AutoGearClamp"(TRUE ("DTResetEncoder")) -> ()
        }
        frame #6 {
          n357 = global write "Robot Global Data.vi" "AutoHopperPanelPistons"(TRUE ("GyroReset")) -> ()
          n358 = global write "Robot Global Data.vi" "AutoStep"("Turn -60" ("AutoStep")) -> ()
          n359 = global write "Robot Global Data.vi" "AutoAngle"(60.0 ("DriveAngle")) -> ()
          n360 = global write "Robot Global Data.vi" "FwdPIDOn"(TRUE ("FwdPIDOn")) -> ()
          n361 = global write "Robot Global Data.vi" "AutoDistance"(-238.0 ("DriveDistance")) -> ()
          n362 = global write "Robot Global Data.vi" "AutoConv+Upt"(FALSE ("DTResetEncoder")) -> ()
          n363 = global write "Robot Global Data.vi" "AutoGyroReset"(FALSE ("GyroReset")) -> ()
          n364 = global write "Robot Global Data.vi" "AutoBallIntake"(TRUE ("DTResetEncoder")) -> ()
          n365 = global write "Robot Global Data.vi" "DTResetEncoder"(FALSE ("DTResetEncoder")) -> ()
          n366 = global write "Robot Global Data.vi" "AutoAngle PIDOn"(TRUE ("AnglePIDOn")) -> ()
          n367 = global write "Robot Global Data.vi" "AutoGearClamp"(TRUE ("DTResetEncoder")) -> ()
          n368 = global write "Robot Global Data.vi" "AutoFlyw"(FALSE ("DTResetEncoder")) -> ()
          n369 = Wait (ms)(milliseconds to wait=u32 1000) -> ()  [unwired: 1 out]
        }
        frame #7 {
          # "-1429"
          n370 = global write "Robot Global Data.vi" "AutoHopperPanelPistons"(TRUE ("GyroReset")) -> ()
          n371 = global write "Robot Global Data.vi" "AutoStep"("Backup" ("AutoStep")) -> ()
          n372 = global write "Robot Global Data.vi" "AutoAngle"(60.0 ("DriveAngle")) -> ()
          n373 = global write "Robot Global Data.vi" "FwdPIDOn"(TRUE ("FwdPIDOn")) -> ()
          n374 = global write "Robot Global Data.vi" "AutoDistance"(-4287.0 ("DriveDistance")) -> ()
          n375 = global write "Robot Global Data.vi" "AutoConv+Upt"(FALSE ("DTResetEncoder")) -> ()
          n376 = global write "Robot Global Data.vi" "AutoGyroReset"(FALSE ("GyroReset")) -> ()
          n377 = global write "Robot Global Data.vi" "AutoBallIntake"(TRUE ("DTResetEncoder")) -> ()
          n378 = global write "Robot Global Data.vi" "DTResetEncoder"(FALSE ("DTResetEncoder")) -> ()
          n379 = global write "Robot Global Data.vi" "AutoAngle PIDOn"(TRUE ("AnglePIDOn")) -> ()
          n380 = global write "Robot Global Data.vi" "AutoGearClamp"(TRUE ("DTResetEncoder")) -> ()
          n381 = global write "Robot Global Data.vi" "AutoFlyw"(FALSE ("DTResetEncoder")) -> ()
          n382 = Wait (ms)(milliseconds to wait=u32 3000) -> ()  [unwired: 1 out]
        }
        frame #8 {
          n383 = global write "Robot Global Data.vi" "AutoHopperPanelPistons"(TRUE ("GyroReset")) -> ()
          n384 = global write "Robot Global Data.vi" "AutoGearClamp"(TRUE ("DTResetEncoder")) -> ()
          n385 = global write "Robot Global Data.vi" "AutoStep"("reset+stop" ("AutoStep")) -> ()
          n386 = global write "Robot Global Data.vi" "AutoAngle"(0.0 ("DriveAngle")) -> ()
          n387 = global write "Robot Global Data.vi" "FwdPIDOn"(FALSE ("FwdPIDOn")) -> ()
          n388 = global write "Robot Global Data.vi" "AutoDistance"(0.0 ("DriveDistance")) -> ()
          n389 = global write "Robot Global Data.vi" "AutoGyroReset"(FALSE ("GyroReset")) -> ()
          n390 = global write "Robot Global Data.vi" "DTResetEncoder"(FALSE ("DTResetEncoder")) -> ()
          n391 = global write "Robot Global Data.vi" "AutoAngle PIDOn"(FALSE ("AnglePIDOn")) -> ()
          n392 = global write "Robot Global Data.vi" "AutoConv+Upt"(FALSE ("DTResetEncoder")) -> ()
          n393 = global write "Robot Global Data.vi" "AutoBallIntake"(FALSE ("DTResetEncoder")) -> ()
          n394 = global write "Robot Global Data.vi" "AutoFlyw"(FALSE ("DTResetEncoder")) -> ()
          n395 = Wait (ms)(milliseconds to wait=u32 500) -> ()  [unwired: 1 out]
        }
      }
    }
    frame "V2 Left Peg" {
      n396 = flat-sequence {
        frame #0 {
          n397 = global write "Robot Global Data.vi" "AutoHopperPanelPistons"(FALSE ("GyroReset")) -> ()
          n398 = global write "Robot Global Data.vi" "AutoIntakePistons"(FALSE ("GyroReset")) -> ()
          n399 = global write "Robot Global Data.vi" "AutoStep"("start" ("AutoStep")) -> ()
          n400 = global write "Robot Global Data.vi" "FwdPIDOn"(FALSE ("FwdPIDOn")) -> ()
          n401 = global write "Robot Global Data.vi" "DriveAngle"(0.0 ("DriveAngle")) -> ()
          n402 = global write "Robot Global Data.vi" "AutoGearClamp"(TRUE ("DTResetEncoder")) -> ()
          n403 = global write "Robot Global Data.vi" "DriveDistance"(0.0 ("DriveDistance")) -> ()
          n404 = global write "Robot Global Data.vi" "AutoGyroReset"(FALSE ("GyroReset")) -> ()
          n405 = global write "Robot Global Data.vi" "DTResetEncoder"(FALSE ("DTResetEncoder")) -> ()
          n406 = global write "Robot Global Data.vi" "AutoAngle PIDOn"(FALSE ("AnglePIDOn")) -> ()
          n407 = Wait (ms)(milliseconds to wait=u32 20) -> ()  [unwired: 1 out]
        }
        frame #1 {
          n408 = global write "Robot Global Data.vi" "AutoHopperPanelPistons"(FALSE ("GyroReset")) -> ()
          n409 = global write "Robot Global Data.vi" "AutoIntakePistons"(FALSE ("GyroReset")) -> ()
          n410 = global write "Robot Global Data.vi" "AutoStep"("reset+spoiler up" ("AutoStep")) -> ()
          n411 = global write "Robot Global Data.vi" "AutoAngle"(0.0 ("DriveAngle")) -> ()
          n412 = global write "Robot Global Data.vi" "FwdPIDOn"(FALSE ("FwdPIDOn")) -> ()
          n413 = global write "Robot Global Data.vi" "AutoDistance"(0.0 ("DriveDistance")) -> ()
          n414 = global write "Robot Global Data.vi" "AutoGearClamp"(TRUE ("DTResetEncoder")) -> ()
          n415 = global write "Robot Global Data.vi" "AutoGyroReset"(TRUE ("GyroReset")) -> ()
          n416 = global write "Robot Global Data.vi" "DTResetEncoder"(TRUE ("DTResetEncoder")) -> ()
          n417 = global write "Robot Global Data.vi" "AutoAngle PIDOn"(FALSE ("AnglePIDOn")) -> ()
          n418 = Wait (ms)(milliseconds to wait=u32 500) -> ()  [unwired: 1 out]
        }
        frame #2 {
          n419 = global write "Robot Global Data.vi" "AutoHopperPanelPistons"(TRUE ("GyroReset")) -> ()
          n420 = global write "Robot Global Data.vi" "AutoIntakePistons"(FALSE ("GyroReset")) -> ()
          n421 = global write "Robot Global Data.vi" "AutoStep"("PID on" ("AutoStep")) -> ()
          n422 = global write "Robot Global Data.vi" "AutoAngle"(0.0 ("DriveAngle")) -> ()
          n423 = global write "Robot Global Data.vi" "FwdPIDOn"(TRUE ("FwdPIDOn")) -> ()
          n424 = global write "Robot Global Data.vi" "AutoDistance"(0.0 ("DriveDistance")) -> ()
          n425 = global write "Robot Global Data.vi" "AutoGearClamp"(TRUE ("DTResetEncoder")) -> ()
          n426 = global write "Robot Global Data.vi" "AutoGyroReset"(FALSE ("GyroReset")) -> ()
          n427 = global write "Robot Global Data.vi" "DTResetEncoder"(FALSE ("DTResetEncoder")) -> ()
          n428 = global write "Robot Global Data.vi" "AutoAngle PIDOn"(TRUE ("AnglePIDOn")) -> ()
          n429 = Wait (ms)(milliseconds to wait=u32 300) -> ()  [unwired: 1 out]
        }
        frame #3 {
          # "xx"
          n430 = global write "Robot Global Data.vi" "AutoHopperPanelPistons"(TRUE ("GyroReset")) -> ()
          n431 = global write "Robot Global Data.vi" "AutoIntakePistons"(FALSE ("GyroReset")) -> ()
          n432 = global write "Robot Global Data.vi" "AutoStep"("drive fwd" ("AutoStep")) -> ()
          n433 = global write "Robot Global Data.vi" "AutoAngle"(0.0 ("DriveAngle")) -> ()
          n434 = global write "Robot Global Data.vi" "FwdPIDOn"(TRUE ("FwdPIDOn")) -> ()
          n435 = global write "Robot Global Data.vi" "AutoDistance"(3668.0 ("DriveDistance")) -> ()
          n436 = global write "Robot Global Data.vi" "AutoGearClamp"(TRUE ("DTResetEncoder")) -> ()
          n437 = global write "Robot Global Data.vi" "AutoGyroReset"(FALSE ("GyroReset")) -> ()
          n438 = global write "Robot Global Data.vi" "DTResetEncoder"(FALSE ("DTResetEncoder")) -> ()
          n439 = global write "Robot Global Data.vi" "AutoAngle PIDOn"(TRUE ("AnglePIDOn")) -> ()
          n440 = Wait (ms)(milliseconds to wait=u32 3000) -> ()  [unwired: 1 out]
        }
        frame #4 {
          n441 = global write "Robot Global Data.vi" "AutoHopperPanelPistons"(TRUE ("GyroReset")) -> ()
          n442 = global write "Robot Global Data.vi" "AutoIntakePistons"(FALSE ("GyroReset")) -> ()
          n443 = global write "Robot Global Data.vi" "AutoStep"("Fwd PID Off " ("AutoStep")) -> ()
          n444 = global write "Robot Global Data.vi" "AutoAngle"(0.0 ("DriveAngle")) -> ()
          n445 = global write "Robot Global Data.vi" "FwdPIDOn"(FALSE ("FwdPIDOn")) -> ()
          n446 = global write "Robot Global Data.vi" "AutoDistance"(3668.0 ("DriveDistance")) -> ()
          n447 = global write "Robot Global Data.vi" "AutoGearClamp"(TRUE ("DTResetEncoder")) -> ()
          n448 = global write "Robot Global Data.vi" "AutoGyroReset"(FALSE ("GyroReset")) -> ()
          n449 = global write "Robot Global Data.vi" "DTResetEncoder"(FALSE ("DTResetEncoder")) -> ()
          n450 = global write "Robot Global Data.vi" "AutoAngle PIDOn"(TRUE ("AnglePIDOn")) -> ()
          n451 = Wait (ms)(milliseconds to wait=u32 100) -> ()  [unwired: 1 out]
        }
        frame #5 {
          n452 = global write "Robot Global Data.vi" "AutoHopperPanelPistons"(TRUE ("GyroReset")) -> ()
          n453 = global write "Robot Global Data.vi" "AutoIntakePistons"(FALSE ("GyroReset")) -> ()
          n454 = global write "Robot Global Data.vi" "AutoStep"("Turn Right" ("AutoStep")) -> ()
          n455 = global write "Robot Global Data.vi" "AutoAngle"(60.0 ("DriveAngle")) -> ()
          n456 = global write "Robot Global Data.vi" "FwdPIDOn"(FALSE ("FwdPIDOn")) -> ()
          n457 = global write "Robot Global Data.vi" "AutoDistance"(0.0 ("DriveDistance")) -> ()
          n458 = global write "Robot Global Data.vi" "AutoGearClamp"(TRUE ("DTResetEncoder")) -> ()
          n459 = global write "Robot Global Data.vi" "AutoGyroReset"(FALSE ("GyroReset")) -> ()
          n460 = global write "Robot Global Data.vi" "DTResetEncoder"(FALSE ("DTResetEncoder")) -> ()
          n461 = global write "Robot Global Data.vi" "AutoAngle PIDOn"(TRUE ("AnglePIDOn")) -> ()
          n462 = Wait (ms)(milliseconds to wait=u32 2000) -> ()  [unwired: 1 out]
        }
        frame #6 {
          n463 = global write "Robot Global Data.vi" "AutoHopperPanelPistons"(TRUE ("GyroReset")) -> ()
          n464 = global write "Robot Global Data.vi" "AutoIntakePistons"(FALSE ("GyroReset")) -> ()
          n465 = global write "Robot Global Data.vi" "AutoStep"("Reset Encoders " ("AutoStep")) -> ()
          n466 = global write "Robot Global Data.vi" "AutoAngle"(60.0 ("DriveAngle")) -> ()
          n467 = global write "Robot Global Data.vi" "FwdPIDOn"(FALSE ("FwdPIDOn")) -> ()
          n468 = global write "Robot Global Data.vi" "AutoDistance"(0.0 ("DriveDistance")) -> ()
          n469 = global write "Robot Global Data.vi" "AutoGearClamp"(TRUE ("DTResetEncoder")) -> ()
          n470 = global write "Robot Global Data.vi" "AutoGyroReset"(FALSE ("GyroReset")) -> ()
          n471 = global write "Robot Global Data.vi" "DTResetEncoder"(TRUE ("DTResetEncoder")) -> ()
          n472 = global write "Robot Global Data.vi" "AutoAngle PIDOn"(TRUE ("AnglePIDOn")) -> ()
          n473 = Wait (ms)(milliseconds to wait=u32 500) -> ()  [unwired: 1 out]
        }
        frame #7 {
          # "xx\""
          n474 = global write "Robot Global Data.vi" "AutoHopperPanelPistons"(TRUE ("GyroReset")) -> ()
          n475 = global write "Robot Global Data.vi" "AutoIntakePistons"(FALSE ("GyroReset")) -> ()
          n476 = global write "Robot Global Data.vi" "AutoStep"("drive fwd after turn" ("AutoStep")) -> ()
          n477 = global write "Robot Global Data.vi" "AutoAngle"(60.0 ("DriveAngle")) -> ()
          n478 = global write "Robot Global Data.vi" "FwdPIDOn"(TRUE ("FwdPIDOn")) -> ()
          n479 = global write "Robot Global Data.vi" "AutoDistance"(1338.0 ("DriveDistance")) -> ()
          n480 = global write "Robot Global Data.vi" "AutoGearClamp"(TRUE ("DTResetEncoder")) -> ()
          n481 = global write "Robot Global Data.vi" "AutoGyroReset"(FALSE ("GyroReset")) -> ()
          n482 = global write "Robot Global Data.vi" "DTResetEncoder"(FALSE ("DTResetEncoder")) -> ()
          n483 = global write "Robot Global Data.vi" "AutoAngle PIDOn"(TRUE ("AnglePIDOn")) -> ()
          n484 = Wait (ms)(milliseconds to wait=u32 2500) -> ()  [unwired: 1 out]
        }
        frame #8 {
          n485 = global write "Robot Global Data.vi" "AutoHopperPanelPistons"(TRUE ("GyroReset")) -> ()
          n486 = global write "Robot Global Data.vi" "AutoIntakePistons"(FALSE ("GyroReset")) -> ()
          n487 = global write "Robot Global Data.vi" "AutoStep"("open gear clamp" ("AutoStep")) -> ()
          n488 = global write "Robot Global Data.vi" "AutoAngle"(60.0 ("DriveAngle")) -> ()
          n489 = global write "Robot Global Data.vi" "FwdPIDOn"(TRUE ("FwdPIDOn")) -> ()
          n490 = global write "Robot Global Data.vi" "AutoDistance"(1338.0 ("DriveDistance")) -> ()
          n491 = global write "Robot Global Data.vi" "AutoGearClamp"(FALSE ("DTResetEncoder")) -> ()
          n492 = global write "Robot Global Data.vi" "AutoGyroReset"(FALSE ("GyroReset")) -> ()
          n493 = global write "Robot Global Data.vi" "DTResetEncoder"(FALSE ("DTResetEncoder")) -> ()
          n494 = global write "Robot Global Data.vi" "AutoAngle PIDOn"(TRUE ("AnglePIDOn")) -> ()
          n495 = Wait (ms)(milliseconds to wait=u32 500) -> ()  [unwired: 1 out]
        }
        frame #9 {
          # "0\""
          n496 = global write "Robot Global Data.vi" "AutoHopperPanelPistons"(TRUE ("GyroReset")) -> ()
          n497 = global write "Robot Global Data.vi" "AutoIntakePistons"(TRUE ("GyroReset")) -> ()
          n498 = global write "Robot Global Data.vi" "AutoStep"("drive back + intake down" ("AutoStep")) -> ()
          n499 = global write "Robot Global Data.vi" "AutoAngle"(60.0 ("DriveAngle")) -> ()
          n500 = global write "Robot Global Data.vi" "FwdPIDOn"(TRUE ("FwdPIDOn")) -> ()
          n501 = global write "Robot Global Data.vi" "AutoDistance"(0.0 ("DriveDistance")) -> ()
          n502 = global write "Robot Global Data.vi" "AutoGearClamp"(FALSE ("DTResetEncoder")) -> ()
          n503 = global write "Robot Global Data.vi" "AutoGyroReset"(FALSE ("GyroReset")) -> ()
          n504 = global write "Robot Global Data.vi" "DTResetEncoder"(FALSE ("DTResetEncoder")) -> ()
          n505 = global write "Robot Global Data.vi" "AutoAngle PIDOn"(TRUE ("AnglePIDOn")) -> ()
          n506 = Wait (ms)(milliseconds to wait=u32 2000) -> ()  [unwired: 1 out]
        }
        frame #10 {
          n507 = global write "Robot Global Data.vi" "AutoHopperPanelPistons"(TRUE ("GyroReset")) -> ()
          n508 = global write "Robot Global Data.vi" "AutoIntakePistons"(FALSE ("GyroReset")) -> ()
          n509 = global write "Robot Global Data.vi" "AutoStep"("PIDs Off + Intake up " ("AutoStep")) -> ()
          n510 = global write "Robot Global Data.vi" "AutoAngle"(60.0 ("DriveAngle")) -> ()
          n511 = global write "Robot Global Data.vi" "FwdPIDOn"(FALSE ("FwdPIDOn")) -> ()
          n512 = global write "Robot Global Data.vi" "AutoDistance"(0.0 ("DriveDistance")) -> ()
          n513 = global write "Robot Global Data.vi" "AutoGearClamp"(FALSE ("DTResetEncoder")) -> ()
          n514 = global write "Robot Global Data.vi" "AutoGyroReset"(FALSE ("GyroReset")) -> ()
          n515 = global write "Robot Global Data.vi" "DTResetEncoder"(FALSE ("DTResetEncoder")) -> ()
          n516 = global write "Robot Global Data.vi" "AutoAngle PIDOn"(FALSE ("AnglePIDOn")) -> ()
          n517 = Wait (ms)(milliseconds to wait=u32 1000) -> ()  [unwired: 1 out]
        }
        frame #11 {
          n518 = global write "Robot Global Data.vi" "AutoHopperPanelPistons"(TRUE ("GyroReset")) -> ()
          n519 = global write "Robot Global Data.vi" "AutoIntakePistons"(FALSE ("GyroReset")) -> ()
          n520 = global write "Robot Global Data.vi" "AutoStep"("reset+stop" ("AutoStep")) -> ()
          n521 = global write "Robot Global Data.vi" "AutoAngle"(0.0 ("DriveAngle")) -> ()
          n522 = global write "Robot Global Data.vi" "FwdPIDOn"(FALSE ("FwdPIDOn")) -> ()
          n523 = global write "Robot Global Data.vi" "AutoDistance"(0.0 ("DriveDistance")) -> ()
          n524 = global write "Robot Global Data.vi" "AutoGearClamp"(FALSE ("DTResetEncoder")) -> ()
          n525 = global write "Robot Global Data.vi" "AutoGyroReset"(TRUE ("GyroReset")) -> ()
          n526 = global write "Robot Global Data.vi" "DTResetEncoder"(TRUE ("DTResetEncoder")) -> ()
          n527 = global write "Robot Global Data.vi" "AutoAngle PIDOn"(FALSE ("AnglePIDOn")) -> ()
          n528 = Wait (ms)(milliseconds to wait=u32 500) -> ()  [unwired: 1 out]
        }
        frame #12 {
          n529 = global write "Robot Global Data.vi" "AutoHopperPanelPistons"(TRUE ("GyroReset")) -> ()
          n530 = global write "Robot Global Data.vi" "AutoIntakePistons"(FALSE ("GyroReset")) -> ()
          n531 = global write "Robot Global Data.vi" "AutoStep"("stop" ("AutoStep")) -> ()
          n532 = global write "Robot Global Data.vi" "AutoAngle"(0.0 ("DriveAngle")) -> ()
          n533 = global write "Robot Global Data.vi" "FwdPIDOn"(FALSE ("FwdPIDOn")) -> ()
          n534 = global write "Robot Global Data.vi" "AutoDistance"(0.0 ("DriveDistance")) -> ()
          n535 = global write "Robot Global Data.vi" "AutoGearClamp"(FALSE ("DTResetEncoder")) -> ()
          n536 = global write "Robot Global Data.vi" "AutoGyroReset"(FALSE ("GyroReset")) -> ()
          n537 = global write "Robot Global Data.vi" "DTResetEncoder"(FALSE ("DTResetEncoder")) -> ()
          n538 = global write "Robot Global Data.vi" "AutoAngle PIDOn"(FALSE ("AnglePIDOn")) -> ()
          n539 = Wait (ms)(milliseconds to wait=u32 500) -> ()  [unwired: 1 out]
        }
      }
    }
    frame "V2 Right Peg" {
      n540 = flat-sequence {
        frame #0 {
          n541 = global write "Robot Global Data.vi" "AutoHopperPanelPistons"(FALSE ("GyroReset")) -> ()
          n542 = global write "Robot Global Data.vi" "AutoIntakePistons"(FALSE ("GyroReset")) -> ()
          n543 = global write "Robot Global Data.vi" "AutoStep"("start" ("AutoStep")) -> ()
          n544 = global write "Robot Global Data.vi" "FwdPIDOn"(FALSE ("FwdPIDOn")) -> ()
          n545 = global write "Robot Global Data.vi" "DriveAngle"(0.0 ("DriveAngle")) -> ()
          n546 = global write "Robot Global Data.vi" "AutoGearClamp"(TRUE ("DTResetEncoder")) -> ()
          n547 = global write "Robot Global Data.vi" "DriveDistance"(0.0 ("DriveDistance")) -> ()
          n548 = global write "Robot Global Data.vi" "AutoGyroReset"(FALSE ("GyroReset")) -> ()
          n549 = global write "Robot Global Data.vi" "DTResetEncoder"(FALSE ("DTResetEncoder")) -> ()
          n550 = global write "Robot Global Data.vi" "AutoAngle PIDOn"(FALSE ("AnglePIDOn")) -> ()
          n551 = Wait (ms)(milliseconds to wait=u32 20) -> ()  [unwired: 1 out]
        }
        frame #1 {
          n552 = global write "Robot Global Data.vi" "AutoHopperPanelPistons"(FALSE ("GyroReset")) -> ()
          n553 = global write "Robot Global Data.vi" "AutoIntakePistons"(FALSE ("GyroReset")) -> ()
          n554 = global write "Robot Global Data.vi" "AutoStep"("reset+hopper out" ("AutoStep")) -> ()
          n555 = global write "Robot Global Data.vi" "AutoAngle"(0.0 ("DriveAngle")) -> ()
          n556 = global write "Robot Global Data.vi" "FwdPIDOn"(FALSE ("FwdPIDOn")) -> ()
          n557 = global write "Robot Global Data.vi" "AutoDistance"(0.0 ("DriveDistance")) -> ()
          n558 = global write "Robot Global Data.vi" "AutoGearClamp"(TRUE ("DTResetEncoder")) -> ()
          n559 = global write "Robot Global Data.vi" "AutoGyroReset"(TRUE ("GyroReset")) -> ()
          n560 = global write "Robot Global Data.vi" "DTResetEncoder"(TRUE ("DTResetEncoder")) -> ()
          n561 = global write "Robot Global Data.vi" "AutoAngle PIDOn"(FALSE ("AnglePIDOn")) -> ()
          n562 = Wait (ms)(milliseconds to wait=u32 500) -> ()  [unwired: 1 out]
        }
        frame #2 {
          n563 = global write "Robot Global Data.vi" "AutoHopperPanelPistons"(TRUE ("GyroReset")) -> ()
          n564 = global write "Robot Global Data.vi" "AutoIntakePistons"(FALSE ("GyroReset")) -> ()
          n565 = global write "Robot Global Data.vi" "AutoStep"("PID on" ("AutoStep")) -> ()
          n566 = global write "Robot Global Data.vi" "AutoAngle"(0.0 ("DriveAngle")) -> ()
          n567 = global write "Robot Global Data.vi" "FwdPIDOn"(TRUE ("FwdPIDOn")) -> ()
          n568 = global write "Robot Global Data.vi" "AutoDistance"(0.0 ("DriveDistance")) -> ()
          n569 = global write "Robot Global Data.vi" "AutoGearClamp"(TRUE ("DTResetEncoder")) -> ()
          n570 = global write "Robot Global Data.vi" "AutoGyroReset"(FALSE ("GyroReset")) -> ()
          n571 = global write "Robot Global Data.vi" "DTResetEncoder"(FALSE ("DTResetEncoder")) -> ()
          n572 = global write "Robot Global Data.vi" "AutoAngle PIDOn"(TRUE ("AnglePIDOn")) -> ()
          n573 = Wait (ms)(milliseconds to wait=u32 300) -> ()  [unwired: 1 out]
        }
        frame #3 {
          n574 = global write "Robot Global Data.vi" "AutoHopperPanelPistons"(TRUE ("GyroReset")) -> ()
          n575 = global write "Robot Global Data.vi" "AutoIntakePistons"(FALSE ("GyroReset")) -> ()
          n576 = global write "Robot Global Data.vi" "AutoStep"("drive fwd" ("AutoStep")) -> ()
          n577 = global write "Robot Global Data.vi" "AutoAngle"(0.0 ("DriveAngle")) -> ()
          n578 = global write "Robot Global Data.vi" "FwdPIDOn"(TRUE ("FwdPIDOn")) -> ()
          n579 = global write "Robot Global Data.vi" "AutoDistance"(3468.0 ("DriveDistance")) -> ()
          n580 = global write "Robot Global Data.vi" "AutoGearClamp"(TRUE ("DTResetEncoder")) -> ()
          n581 = global write "Robot Global Data.vi" "AutoGyroReset"(FALSE ("GyroReset")) -> ()
          n582 = global write "Robot Global Data.vi" "DTResetEncoder"(FALSE ("DTResetEncoder")) -> ()
          n583 = global write "Robot Global Data.vi" "AutoAngle PIDOn"(TRUE ("AnglePIDOn")) -> ()
          n584 = Wait (ms)(milliseconds to wait=u32 3000) -> ()  [unwired: 1 out]
        }
        frame #4 {
          n585 = global write "Robot Global Data.vi" "AutoHopperPanelPistons"(TRUE ("GyroReset")) -> ()
          n586 = global write "Robot Global Data.vi" "AutoIntakePistons"(FALSE ("GyroReset")) -> ()
          n587 = global write "Robot Global Data.vi" "AutoStep"("Fwd PID Off " ("AutoStep")) -> ()
          n588 = global write "Robot Global Data.vi" "AutoAngle"(0.0 ("DriveAngle")) -> ()
          n589 = global write "Robot Global Data.vi" "FwdPIDOn"(FALSE ("FwdPIDOn")) -> ()
          n590 = global write "Robot Global Data.vi" "AutoDistance"(3468.0 ("DriveDistance")) -> ()
          n591 = global write "Robot Global Data.vi" "AutoGearClamp"(TRUE ("DTResetEncoder")) -> ()
          n592 = global write "Robot Global Data.vi" "AutoGyroReset"(FALSE ("GyroReset")) -> ()
          n593 = global write "Robot Global Data.vi" "DTResetEncoder"(FALSE ("DTResetEncoder")) -> ()
          n594 = global write "Robot Global Data.vi" "AutoAngle PIDOn"(TRUE ("AnglePIDOn")) -> ()
          n595 = Wait (ms)(milliseconds to wait=u32 100) -> ()  [unwired: 1 out]
        }
        frame #5 {
          n596 = global write "Robot Global Data.vi" "AutoHopperPanelPistons"(TRUE ("GyroReset")) -> ()
          n597 = global write "Robot Global Data.vi" "AutoIntakePistons"(FALSE ("GyroReset")) -> ()
          n598 = global write "Robot Global Data.vi" "AutoStep"("Turn Right" ("AutoStep")) -> ()
          n599 = global write "Robot Global Data.vi" "AutoAngle"(-60.0 ("DriveAngle")) -> ()
          n600 = global write "Robot Global Data.vi" "FwdPIDOn"(FALSE ("FwdPIDOn")) -> ()
          n601 = global write "Robot Global Data.vi" "AutoDistance"(0.0 ("DriveDistance")) -> ()
          n602 = global write "Robot Global Data.vi" "AutoGearClamp"(TRUE ("DTResetEncoder")) -> ()
          n603 = global write "Robot Global Data.vi" "AutoGyroReset"(FALSE ("GyroReset")) -> ()
          n604 = global write "Robot Global Data.vi" "DTResetEncoder"(FALSE ("DTResetEncoder")) -> ()
          n605 = global write "Robot Global Data.vi" "AutoAngle PIDOn"(TRUE ("AnglePIDOn")) -> ()
          n606 = Wait (ms)(milliseconds to wait=u32 2000) -> ()  [unwired: 1 out]
        }
        frame #6 {
          n607 = global write "Robot Global Data.vi" "AutoHopperPanelPistons"(TRUE ("GyroReset")) -> ()
          n608 = global write "Robot Global Data.vi" "AutoIntakePistons"(FALSE ("GyroReset")) -> ()
          n609 = global write "Robot Global Data.vi" "AutoStep"("Reset Encoders " ("AutoStep")) -> ()
          n610 = global write "Robot Global Data.vi" "AutoAngle"(-60.0 ("DriveAngle")) -> ()
          n611 = global write "Robot Global Data.vi" "FwdPIDOn"(FALSE ("FwdPIDOn")) -> ()
          n612 = global write "Robot Global Data.vi" "AutoDistance"(0.0 ("DriveDistance")) -> ()
          n613 = global write "Robot Global Data.vi" "AutoGearClamp"(TRUE ("DTResetEncoder")) -> ()
          n614 = global write "Robot Global Data.vi" "AutoGyroReset"(FALSE ("GyroReset")) -> ()
          n615 = global write "Robot Global Data.vi" "DTResetEncoder"(TRUE ("DTResetEncoder")) -> ()
          n616 = global write "Robot Global Data.vi" "AutoAngle PIDOn"(TRUE ("AnglePIDOn")) -> ()
          n617 = Wait (ms)(milliseconds to wait=u32 500) -> ()  [unwired: 1 out]
        }
        frame #7 {
          # "xx\""
          n618 = global write "Robot Global Data.vi" "AutoHopperPanelPistons"(TRUE ("GyroReset")) -> ()
          n619 = global write "Robot Global Data.vi" "AutoIntakePistons"(FALSE ("GyroReset")) -> ()
          n620 = global write "Robot Global Data.vi" "AutoStep"("drive fwd after turn" ("AutoStep")) -> ()
          n621 = global write "Robot Global Data.vi" "AutoAngle"(-60.0 ("DriveAngle")) -> ()
          n622 = global write "Robot Global Data.vi" "FwdPIDOn"(TRUE ("FwdPIDOn")) -> ()
          n623 = global write "Robot Global Data.vi" "AutoDistance"(1378.0 ("DriveDistance")) -> ()
          n624 = global write "Robot Global Data.vi" "AutoGearClamp"(TRUE ("DTResetEncoder")) -> ()
          n625 = global write "Robot Global Data.vi" "AutoGyroReset"(FALSE ("GyroReset")) -> ()
          n626 = global write "Robot Global Data.vi" "DTResetEncoder"(FALSE ("DTResetEncoder")) -> ()
          n627 = global write "Robot Global Data.vi" "AutoAngle PIDOn"(TRUE ("AnglePIDOn")) -> ()
          n628 = Wait (ms)(milliseconds to wait=u32 2500) -> ()  [unwired: 1 out]
        }
        frame #8 {
          n629 = global write "Robot Global Data.vi" "AutoHopperPanelPistons"(TRUE ("GyroReset")) -> ()
          n630 = global write "Robot Global Data.vi" "AutoIntakePistons"(FALSE ("GyroReset")) -> ()
          n631 = global write "Robot Global Data.vi" "AutoStep"("open gear clamp" ("AutoStep")) -> ()
          n632 = global write "Robot Global Data.vi" "AutoAngle"(-60.0 ("DriveAngle")) -> ()
          n633 = global write "Robot Global Data.vi" "FwdPIDOn"(TRUE ("FwdPIDOn")) -> ()
          n634 = global write "Robot Global Data.vi" "AutoDistance"(1378.0 ("DriveDistance")) -> ()
          n635 = global write "Robot Global Data.vi" "AutoGearClamp"(FALSE ("DTResetEncoder")) -> ()
          n636 = global write "Robot Global Data.vi" "AutoGyroReset"(FALSE ("GyroReset")) -> ()
          n637 = global write "Robot Global Data.vi" "DTResetEncoder"(FALSE ("DTResetEncoder")) -> ()
          n638 = global write "Robot Global Data.vi" "AutoAngle PIDOn"(TRUE ("AnglePIDOn")) -> ()
          n639 = Wait (ms)(milliseconds to wait=u32 500) -> ()  [unwired: 1 out]
        }
        frame #9 {
          # "0\""
          n640 = global write "Robot Global Data.vi" "AutoHopperPanelPistons"(TRUE ("GyroReset")) -> ()
          n641 = global write "Robot Global Data.vi" "AutoIntakePistons"(TRUE ("GyroReset")) -> ()
          n642 = global write "Robot Global Data.vi" "AutoStep"("drive back + intake down" ("AutoStep")) -> ()
          n643 = global write "Robot Global Data.vi" "AutoAngle"(-60.0 ("DriveAngle")) -> ()
          n644 = global write "Robot Global Data.vi" "FwdPIDOn"(TRUE ("FwdPIDOn")) -> ()
          n645 = global write "Robot Global Data.vi" "AutoDistance"(0.0 ("DriveDistance")) -> ()
          n646 = global write "Robot Global Data.vi" "AutoGearClamp"(FALSE ("DTResetEncoder")) -> ()
          n647 = global write "Robot Global Data.vi" "AutoGyroReset"(FALSE ("GyroReset")) -> ()
          n648 = global write "Robot Global Data.vi" "DTResetEncoder"(FALSE ("DTResetEncoder")) -> ()
          n649 = global write "Robot Global Data.vi" "AutoAngle PIDOn"(TRUE ("AnglePIDOn")) -> ()
          n650 = Wait (ms)(milliseconds to wait=u32 2000) -> ()  [unwired: 1 out]
        }
        frame #10 {
          n651 = global write "Robot Global Data.vi" "AutoHopperPanelPistons"(TRUE ("GyroReset")) -> ()
          n652 = global write "Robot Global Data.vi" "AutoIntakePistons"(FALSE ("GyroReset")) -> ()
          n653 = global write "Robot Global Data.vi" "AutoStep"("PIDs Off + Intake up " ("AutoStep")) -> ()
          n654 = global write "Robot Global Data.vi" "AutoAngle"(-60.0 ("DriveAngle")) -> ()
          n655 = global write "Robot Global Data.vi" "FwdPIDOn"(FALSE ("FwdPIDOn")) -> ()
          n656 = global write "Robot Global Data.vi" "AutoDistance"(0.0 ("DriveDistance")) -> ()
          n657 = global write "Robot Global Data.vi" "AutoGearClamp"(FALSE ("DTResetEncoder")) -> ()
          n658 = global write "Robot Global Data.vi" "AutoGyroReset"(FALSE ("GyroReset")) -> ()
          n659 = global write "Robot Global Data.vi" "DTResetEncoder"(FALSE ("DTResetEncoder")) -> ()
          n660 = global write "Robot Global Data.vi" "AutoAngle PIDOn"(FALSE ("AnglePIDOn")) -> ()
          n661 = Wait (ms)(milliseconds to wait=u32 1000) -> ()  [unwired: 1 out]
        }
        frame #11 {
          n662 = global write "Robot Global Data.vi" "AutoHopperPanelPistons"(TRUE ("GyroReset")) -> ()
          n663 = global write "Robot Global Data.vi" "AutoIntakePistons"(FALSE ("GyroReset")) -> ()
          n664 = global write "Robot Global Data.vi" "AutoStep"("reset+stop" ("AutoStep")) -> ()
          n665 = global write "Robot Global Data.vi" "AutoAngle"(0.0 ("DriveAngle")) -> ()
          n666 = global write "Robot Global Data.vi" "FwdPIDOn"(FALSE ("FwdPIDOn")) -> ()
          n667 = global write "Robot Global Data.vi" "AutoDistance"(0.0 ("DriveDistance")) -> ()
          n668 = global write "Robot Global Data.vi" "AutoGearClamp"(FALSE ("DTResetEncoder")) -> ()
          n669 = global write "Robot Global Data.vi" "AutoGyroReset"(TRUE ("GyroReset")) -> ()
          n670 = global write "Robot Global Data.vi" "DTResetEncoder"(TRUE ("DTResetEncoder")) -> ()
          n671 = global write "Robot Global Data.vi" "AutoAngle PIDOn"(FALSE ("AnglePIDOn")) -> ()
          n672 = Wait (ms)(milliseconds to wait=u32 500) -> ()  [unwired: 1 out]
        }
        frame #12 {
          n673 = global write "Robot Global Data.vi" "AutoHopperPanelPistons"(TRUE ("GyroReset")) -> ()
          n674 = global write "Robot Global Data.vi" "AutoIntakePistons"(FALSE ("GyroReset")) -> ()
          n675 = global write "Robot Global Data.vi" "AutoStep"("stop" ("AutoStep")) -> ()
          n676 = global write "Robot Global Data.vi" "AutoAngle"(0.0 ("DriveAngle")) -> ()
          n677 = global write "Robot Global Data.vi" "FwdPIDOn"(FALSE ("FwdPIDOn")) -> ()
          n678 = global write "Robot Global Data.vi" "AutoDistance"(0.0 ("DriveDistance")) -> ()
          n679 = global write "Robot Global Data.vi" "AutoGearClamp"(FALSE ("DTResetEncoder")) -> ()
          n680 = global write "Robot Global Data.vi" "AutoGyroReset"(FALSE ("GyroReset")) -> ()
          n681 = global write "Robot Global Data.vi" "DTResetEncoder"(FALSE ("DTResetEncoder")) -> ()
          n682 = global write "Robot Global Data.vi" "AutoAngle PIDOn"(FALSE ("AnglePIDOn")) -> ()
          n683 = Wait (ms)(milliseconds to wait=u32 500) -> ()  [unwired: 1 out]
        }
      }
    }
    frame "V2 Mid Peg" {
      n684 = flat-sequence {
        frame #0 {
          n685 = global write "Robot Global Data.vi" "AutoStep"("start" ("AutoStep")) -> ()
          n686 = global write "Robot Global Data.vi" "FwdPIDOn"(FALSE ("FwdPIDOn")) -> ()
          n687 = global write "Robot Global Data.vi" "DriveAngle"(0.0 ("DriveAngle")) -> ()
          n688 = global write "Robot Global Data.vi" "AutoGearClamp"(TRUE ("DTResetEncoder")) -> ()
          n689 = global write "Robot Global Data.vi" "DriveDistance"(0.0 ("DriveDistance")) -> ()
          n690 = global write "Robot Global Data.vi" "AutoGyroReset"(FALSE ("GyroReset")) -> ()
          n691 = global write "Robot Global Data.vi" "AutoIntakePistons"(FALSE ("GyroReset")) -> ()
          n692 = global write "Robot Global Data.vi" "DTResetEncoder"(FALSE ("DTResetEncoder")) -> ()
          n693 = global write "Robot Global Data.vi" "AutoAngle PIDOn"(FALSE ("AnglePIDOn")) -> ()
          n694 = global write "Robot Global Data.vi" "AutoHopperPanelPistons"(FALSE ("GyroReset")) -> ()
          n695 = Wait (ms)(milliseconds to wait=u32 20) -> ()  [unwired: 1 out]
        }
        frame #1 {
          n696 = global write "Robot Global Data.vi" "AutoHopperPanelPistons"(TRUE ("GyroReset")) -> ()
          n697 = global write "Robot Global Data.vi" "AutoStep"("reset+hopper out" ("AutoStep")) -> ()
          n698 = global write "Robot Global Data.vi" "AutoAngle"(0.0 ("DriveAngle")) -> ()
          n699 = global write "Robot Global Data.vi" "FwdPIDOn"(FALSE ("FwdPIDOn")) -> ()
          n700 = global write "Robot Global Data.vi" "AutoDistance"(0.0 ("DriveDistance")) -> ()
          n701 = global write "Robot Global Data.vi" "AutoGearClamp"(TRUE ("DTResetEncoder")) -> ()
          n702 = global write "Robot Global Data.vi" "AutoGyroReset"(TRUE ("GyroReset")) -> ()
          n703 = global write "Robot Global Data.vi" "AutoIntakePistons"(FALSE ("GyroReset")) -> ()
          n704 = global write "Robot Global Data.vi" "DTResetEncoder"(TRUE ("DTResetEncoder")) -> ()
          n705 = global write "Robot Global Data.vi" "AutoAngle PIDOn"(FALSE ("AnglePIDOn")) -> ()
          n706 = Wait (ms)(milliseconds to wait=u32 500) -> ()  [unwired: 1 out]
        }
        frame #2 {
          n707 = global write "Robot Global Data.vi" "AutoHopperPanelPistons"(TRUE ("GyroReset")) -> ()
          n708 = global write "Robot Global Data.vi" "AutoStep"("PID on" ("AutoStep")) -> ()
          n709 = global write "Robot Global Data.vi" "AutoAngle"(0.0 ("DriveAngle")) -> ()
          n710 = global write "Robot Global Data.vi" "FwdPIDOn"(TRUE ("FwdPIDOn")) -> ()
          n711 = global write "Robot Global Data.vi" "AutoDistance"(0.0 ("DriveDistance")) -> ()
          n712 = global write "Robot Global Data.vi" "AutoGearClamp"(TRUE ("DTResetEncoder")) -> ()
          n713 = global write "Robot Global Data.vi" "AutoGyroReset"(FALSE ("GyroReset")) -> ()
          n714 = global write "Robot Global Data.vi" "AutoIntakePistons"(FALSE ("GyroReset")) -> ()
          n715 = global write "Robot Global Data.vi" "DTResetEncoder"(FALSE ("DTResetEncoder")) -> ()
          n716 = global write "Robot Global Data.vi" "AutoAngle PIDOn"(TRUE ("AnglePIDOn")) -> ()
          n717 = Wait (ms)(milliseconds to wait=u32 300) -> ()  [unwired: 1 out]
        }
        frame #3 {
          # "72\""
          # "xx\""
          n718 = global write "Robot Global Data.vi" "AutoHopperPanelPistons"(TRUE ("GyroReset")) -> ()
          n719 = global write "Robot Global Data.vi" "AutoStep"("drive fwd" ("AutoStep")) -> ()
          n720 = global write "Robot Global Data.vi" "AutoAngle"(0.0 ("DriveAngle")) -> ()
          n721 = global write "Robot Global Data.vi" "FwdPIDOn"(TRUE ("FwdPIDOn")) -> ()
          n722 = global write "Robot Global Data.vi" "AutoDistance"(2921.0 ("DriveDistance")) -> ()
          n723 = global write "Robot Global Data.vi" "AutoGearClamp"(TRUE ("DTResetEncoder")) -> ()
          n724 = global write "Robot Global Data.vi" "AutoGyroReset"(FALSE ("GyroReset")) -> ()
          n725 = global write "Robot Global Data.vi" "AutoIntakePistons"(FALSE ("GyroReset")) -> ()
          n726 = global write "Robot Global Data.vi" "DTResetEncoder"(FALSE ("DTResetEncoder")) -> ()
          n727 = global write "Robot Global Data.vi" "AutoAngle PIDOn"(TRUE ("AnglePIDOn")) -> ()
          n728 = Wait (ms)(milliseconds to wait=u32 4000) -> ()  [unwired: 1 out]
        }
        frame #4 {
          n729 = global write "Robot Global Data.vi" "AutoHopperPanelPistons"(TRUE ("GyroReset")) -> ()
          n730 = global write "Robot Global Data.vi" "AutoStep"("open gear clamp" ("AutoStep")) -> ()
          n731 = global write "Robot Global Data.vi" "AutoAngle"(0.0 ("DriveAngle")) -> ()
          n732 = global write "Robot Global Data.vi" "FwdPIDOn"(TRUE ("FwdPIDOn")) -> ()
          n733 = global write "Robot Global Data.vi" "AutoDistance"(2921.0 ("DriveDistance")) -> ()
          n734 = global write "Robot Global Data.vi" "AutoGearClamp"(FALSE ("DTResetEncoder")) -> ()
          n735 = global write "Robot Global Data.vi" "AutoGyroReset"(FALSE ("GyroReset")) -> ()
          n736 = global write "Robot Global Data.vi" "AutoIntakePistons"(FALSE ("GyroReset")) -> ()
          n737 = global write "Robot Global Data.vi" "DTResetEncoder"(FALSE ("DTResetEncoder")) -> ()
          n738 = global write "Robot Global Data.vi" "AutoAngle PIDOn"(TRUE ("AnglePIDOn")) -> ()
          n739 = Wait (ms)(milliseconds to wait=u32 200) -> ()  [unwired: 1 out]
        }
        frame #5 {
          n740 = global write "Robot Global Data.vi" "AutoHopperPanelPistons"(TRUE ("GyroReset")) -> ()
          n741 = global write "Robot Global Data.vi" "AutoStep"("drive back" ("AutoStep")) -> ()
          n742 = global write "Robot Global Data.vi" "AutoAngle"(0.0 ("DriveAngle")) -> ()
          n743 = global write "Robot Global Data.vi" "FwdPIDOn"(TRUE ("FwdPIDOn")) -> ()
          n744 = global write "Robot Global Data.vi" "AutoDistance"(1000.0 ("DriveDistance")) -> ()
          n745 = global write "Robot Global Data.vi" "AutoGearClamp"(FALSE ("DTResetEncoder")) -> ()
          n746 = global write "Robot Global Data.vi" "AutoGyroReset"(FALSE ("GyroReset")) -> ()
          n747 = global write "Robot Global Data.vi" "AutoIntakePistons"(TRUE ("GyroReset")) -> ()
          n748 = global write "Robot Global Data.vi" "DTResetEncoder"(FALSE ("DTResetEncoder")) -> ()
          n749 = global write "Robot Global Data.vi" "AutoAngle PIDOn"(TRUE ("AnglePIDOn")) -> ()
          n750 = Wait (ms)(milliseconds to wait=u32 3000) -> ()  [unwired: 1 out]
        }
        frame #6 {
          n751 = global write "Robot Global Data.vi" "AutoStep"("turn off pid" ("AutoStep")) -> ()
          n752 = global write "Robot Global Data.vi" "AutoAngle"(0.0 ("DriveAngle")) -> ()
          n753 = global write "Robot Global Data.vi" "FwdPIDOn"(FALSE ("FwdPIDOn")) -> ()
          n754 = global write "Robot Global Data.vi" "AutoGearClamp"(FALSE ("DTResetEncoder")) -> ()
          n755 = global write "Robot Global Data.vi" "AutoGyroReset"(FALSE ("GyroReset")) -> ()
          n756 = global write "Robot Global Data.vi" "AutoIntakePistons"(TRUE ("GyroReset")) -> ()
          n757 = global write "Robot Global Data.vi" "AutoHopperPanelPistons"(TRUE ("GyroReset")) -> ()
          n758 = global write "Robot Global Data.vi" "DTResetEncoder"(FALSE ("DTResetEncoder")) -> ()
          n759 = global write "Robot Global Data.vi" "AutoAngle PIDOn"(FALSE ("AnglePIDOn")) -> ()
          n760 = global write "Robot Global Data.vi" "AutoDistance"(1000.0 ("DriveDistance")) -> ()
          n761 = Wait (ms)(milliseconds to wait=u32 500) -> ()  [unwired: 1 out]
        }
        frame #7 {
          n762 = global write "Robot Global Data.vi" "AutoStep"("stop" ("AutoStep")) -> ()
          n763 = global write "Robot Global Data.vi" "AutoAngle"(0.0 ("DriveAngle")) -> ()
          n764 = global write "Robot Global Data.vi" "FwdPIDOn"(FALSE ("FwdPIDOn")) -> ()
          n765 = global write "Robot Global Data.vi" "AutoHopperPanelPistons"(TRUE ("GyroReset")) -> ()
          n766 = global write "Robot Global Data.vi" "AutoDistance"(0.0 ("DriveDistance")) -> ()
          n767 = global write "Robot Global Data.vi" "AutoGearClamp"(FALSE ("DTResetEncoder")) -> ()
          n768 = global write "Robot Global Data.vi" "AutoGyroReset"(FALSE ("GyroReset")) -> ()
          n769 = global write "Robot Global Data.vi" "AutoIntakePistons"(FALSE ("GyroReset")) -> ()
          n770 = global write "Robot Global Data.vi" "DTResetEncoder"(FALSE ("DTResetEncoder")) -> ()
          n771 = global write "Robot Global Data.vi" "AutoAngle PIDOn"(FALSE ("AnglePIDOn")) -> ()
          n772 = Wait (ms)(milliseconds to wait=u32 200) -> ()  [unwired: 1 out]
        }
      }
    }
    frame "Hopper Shoot" {
      n773 = flat-sequence {
        frame #0 {
          n774 = global write "Robot Global Data.vi" "AutoStep"("start" ("AutoStep")) -> ()
          n775 = global write "Robot Global Data.vi" "FwdPIDOn"(FALSE ("FwdPIDOn")) -> ()
          n776 = global write "Robot Global Data.vi" "DriveAngle"(0.0 ("DriveAngle")) -> ()
          n777 = global write "Robot Global Data.vi" "AutoGearClamp"(TRUE ("DTResetEncoder")) -> ()
          n778 = global write "Robot Global Data.vi" "DriveDistance"(0.0 ("DriveDistance")) -> ()
          n779 = global write "Robot Global Data.vi" "AutoGyroReset"(FALSE ("GyroReset")) -> ()
          n780 = global write "Robot Global Data.vi" "AutoIntakePistons"(FALSE ("GyroReset")) -> ()
          n781 = global write "Robot Global Data.vi" "DTResetEncoder"(FALSE ("DTResetEncoder")) -> ()
          n782 = global write "Robot Global Data.vi" "AutoAngle PIDOn"(FALSE ("AnglePIDOn")) -> ()
          n783 = global write "Robot Global Data.vi" "AutoHopperPanelPistons"(FALSE ("GyroReset")) -> ()
          n784 = global write "Robot Global Data.vi" "AutoConv+Upt"(FALSE ("DTResetEncoder")) -> ()
          n785 = global write "Robot Global Data.vi" "AutoFlyw"(FALSE ("DTResetEncoder")) -> ()
          n786 = Wait (ms)(milliseconds to wait=u32 20) -> ()  [unwired: 1 out]
        }
        frame #1 {
          n787 = global write "Robot Global Data.vi" "AutoHopperPanelPistons"(TRUE ("GyroReset")) -> ()
          n788 = global write "Robot Global Data.vi" "AutoStep"("reset+hopper out" ("AutoStep")) -> ()
          n789 = global write "Robot Global Data.vi" "AutoAngle"(0.0 ("DriveAngle")) -> ()
          n790 = global write "Robot Global Data.vi" "FwdPIDOn"(FALSE ("FwdPIDOn")) -> ()
          n791 = global write "Robot Global Data.vi" "AutoDistance"(0.0 ("DriveDistance")) -> ()
          n792 = global write "Robot Global Data.vi" "AutoGearClamp"(TRUE ("DTResetEncoder")) -> ()
          n793 = global write "Robot Global Data.vi" "AutoGyroReset"(TRUE ("GyroReset")) -> ()
          n794 = global write "Robot Global Data.vi" "AutoIntakePistons"(FALSE ("GyroReset")) -> ()
          n795 = global write "Robot Global Data.vi" "DTResetEncoder"(TRUE ("DTResetEncoder")) -> ()
          n796 = global write "Robot Global Data.vi" "AutoAngle PIDOn"(FALSE ("AnglePIDOn")) -> ()
          n797 = global write "Robot Global Data.vi" "AutoBallIntake"(FALSE ("DTResetEncoder")) -> ()
          n798 = global write "Robot Global Data.vi" "AutoFlyw"(FALSE ("DTResetEncoder")) -> ()
          n799 = global write "Robot Global Data.vi" "AutoConv+Upt"(FALSE ("DTResetEncoder")) -> ()
          n800 = Wait (ms)(milliseconds to wait=u32 500) -> ()  [unwired: 1 out]
        }
        frame #2 {
          n801 = global write "Robot Global Data.vi" "AutoHopperPanelPistons"(TRUE ("GyroReset")) -> ()
          n802 = global write "Robot Global Data.vi" "AutoConv+Upt"(FALSE ("DTResetEncoder")) -> ()
          n803 = global write "Robot Global Data.vi" "AutoStep"("PID on" ("AutoStep")) -> ()
          n804 = global write "Robot Global Data.vi" "AutoAngle"(0.0 ("DriveAngle")) -> ()
          n805 = global write "Robot Global Data.vi" "FwdPIDOn"(TRUE ("FwdPIDOn")) -> ()
          n806 = global write "Robot Global Data.vi" "AutoDistance"(0.0 ("DriveDistance")) -> ()
          n807 = global write "Robot Global Data.vi" "AutoGearClamp"(TRUE ("DTResetEncoder")) -> ()
          n808 = global write "Robot Global Data.vi" "AutoGyroReset"(FALSE ("GyroReset")) -> ()
          n809 = global write "Robot Global Data.vi" "AutoIntakePistons"(FALSE ("GyroReset")) -> ()
          n810 = global write "Robot Global Data.vi" "DTResetEncoder"(FALSE ("DTResetEncoder")) -> ()
          n811 = global write "Robot Global Data.vi" "AutoAngle PIDOn"(TRUE ("AnglePIDOn")) -> ()
          n812 = global write "Robot Global Data.vi" "AutoBallIntake"(FALSE ("DTResetEncoder")) -> ()
          n813 = global write "Robot Global Data.vi" "AutoFlyw"(FALSE ("DTResetEncoder")) -> ()
          n814 = Wait (ms)(milliseconds to wait=u32 300) -> ()  [unwired: 1 out]
        }
        frame #3 {
          n815 = global write "Robot Global Data.vi" "AutoHopperPanelPistons"(TRUE ("GyroReset")) -> ()
          n816 = global write "Robot Global Data.vi" "AutoStep"("drive bkwds" ("AutoStep")) -> ()
          n817 = global write "Robot Global Data.vi" "AutoAngle"(0.0 ("DriveAngle")) -> ()
          n818 = global write "Robot Global Data.vi" "FwdPIDOn"(TRUE ("FwdPIDOn")) -> ()
          n819 = global write "Robot Global Data.vi" "AutoDistance"(-5268.0 ("DriveDistance")) -> ()
          n820 = global write "Robot Global Data.vi" "AutoGearClamp"(TRUE ("DTResetEncoder")) -> ()
          n821 = global write "Robot Global Data.vi" "AutoGyroReset"(FALSE ("GyroReset")) -> ()
          n822 = global write "Robot Global Data.vi" "AutoIntakePistons"(FALSE ("GyroReset")) -> ()
          n823 = global write "Robot Global Data.vi" "AutoConv+Upt"(FALSE ("DTResetEncoder")) -> ()
          n824 = global write "Robot Global Data.vi" "DTResetEncoder"(FALSE ("DTResetEncoder")) -> ()
          n825 = global write "Robot Global Data.vi" "AutoAngle PIDOn"(TRUE ("AnglePIDOn")) -> ()
          n826 = global write "Robot Global Data.vi" "AutoBallIntake"(FALSE ("DTResetEncoder")) -> ()
          n827 = global write "Robot Global Data.vi" "AutoFlyw"(FALSE ("DTResetEncoder")) -> ()
          n828 = Wait (ms)(milliseconds to wait=u32 4000) -> ()  [unwired: 1 out]
        }
        frame #4 {
          n829 = global write "Robot Global Data.vi" "AutoHopperPanelPistons"(TRUE ("GyroReset")) -> ()
          n830 = global write "Robot Global Data.vi" "AutoBallIntake"(FALSE ("DTResetEncoder")) -> ()
          n831 = global write "Robot Global Data.vi" "AutoFlyw"(FALSE ("DTResetEncoder")) -> ()
          n832 = global write "Robot Global Data.vi" "AutoStep"("Fwd PID Off " ("AutoStep")) -> ()
          n833 = global write "Robot Global Data.vi" "AutoGearClamp"(TRUE ("DTResetEncoder")) -> ()
          n834 = global write "Robot Global Data.vi" "AutoAngle"(0.0 ("DriveAngle")) -> ()
          n835 = global write "Robot Global Data.vi" "FwdPIDOn"(FALSE ("FwdPIDOn")) -> ()
          n836 = global write "Robot Global Data.vi" "AutoIntakePistons"(FALSE ("GyroReset")) -> ()
          n837 = global write "Robot Global Data.vi" "AutoConv+Upt"(FALSE ("DTResetEncoder")) -> ()
          n838 = global write "Robot Global Data.vi" "AutoDistance"(-5268.0 ("DriveDistance")) -> ()
          n839 = global write "Robot Global Data.vi" "AutoGyroReset"(FALSE ("GyroReset")) -> ()
          n840 = global write "Robot Global Data.vi" "DTResetEncoder"(FALSE ("DTResetEncoder")) -> ()
          n841 = global write "Robot Global Data.vi" "AutoAngle PIDOn"(TRUE ("AnglePIDOn")) -> ()
          n842 = Wait (ms)(milliseconds to wait=u32 100) -> ()  [unwired: 1 out]
        }
        frame #5 {
          n843 = global write "Robot Global Data.vi" "AutoStep"("Turn Right" ("AutoStep")) -> ()
          n844 = global write "Robot Global Data.vi" "AutoAngle"(-60.0 ("DriveAngle")) -> ()
          n845 = global write "Robot Global Data.vi" "FwdPIDOn"(FALSE ("FwdPIDOn")) -> ()
          n846 = global write "Robot Global Data.vi" "AutoDistance"(0.0 ("DriveDistance")) -> ()
          n847 = global write "Robot Global Data.vi" "AutoGyroReset"(FALSE ("GyroReset")) -> ()
          n848 = global write "Robot Global Data.vi" "DTResetEncoder"(FALSE ("DTResetEncoder")) -> ()
          n849 = global write "Robot Global Data.vi" "AutoAngle PIDOn"(TRUE ("AnglePIDOn")) -> ()
          n850 = Wait (ms)(milliseconds to wait=u32 2000) -> ()  [unwired: 1 out]
          n851 = global write "Robot Global Data.vi" "AutoBallIntake"(TRUE ("DTResetEncoder")) -> ()
          n852 = global write "Robot Global Data.vi" "AutoHopperPanelPistons"(TRUE ("GyroReset")) -> ()
          n853 = global write "Robot Global Data.vi" "AutoFlyw"(FALSE ("DTResetEncoder")) -> ()
          n854 = global write "Robot Global Data.vi" "AutoConv+Upt"(FALSE ("DTResetEncoder")) -> ()
          n855 = global write "Robot Global Data.vi" "AutoGearClamp"(TRUE ("DTResetEncoder")) -> ()
          n856 = global write "Robot Global Data.vi" "AutoIntakePistons"(FALSE ("GyroReset")) -> ()
        }
        frame #6 {
          n857 = global write "Robot Global Data.vi" "AutoHopperPanelPistons"(TRUE ("GyroReset")) -> ()
          n858 = global write "Robot Global Data.vi" "AutoStep"("Reset Encoders + gyro " ("AutoStep")) -> ()
          n859 = global write "Robot Global Data.vi" "AutoAngle"(0.0 ("DriveAngle")) -> ()
          n860 = global write "Robot Global Data.vi" "FwdPIDOn"(FALSE ("FwdPIDOn")) -> ()
          n861 = global write "Robot Global Data.vi" "AutoDistance"(0.0 ("DriveDistance")) -> ()
          n862 = global write "Robot Global Data.vi" "AutoGyroReset"(TRUE ("GyroReset")) -> ()
          n863 = global write "Robot Global Data.vi" "DTResetEncoder"(TRUE ("DTResetEncoder")) -> ()
          n864 = global write "Robot Global Data.vi" "AutoAngle PIDOn"(TRUE ("AnglePIDOn")) -> ()
          n865 = global write "Robot Global Data.vi" "AutoGearClamp"(TRUE ("DTResetEncoder")) -> ()
          n866 = global write "Robot Global Data.vi" "AutoIntakePistons"(FALSE ("GyroReset")) -> ()
          n867 = global write "Robot Global Data.vi" "AutoBallIntake"(TRUE ("DTResetEncoder")) -> ()
          n868 = Wait (ms)(milliseconds to wait=u32 500) -> ()  [unwired: 1 out]
          n869 = global write "Robot Global Data.vi" "AutoConv+Upt"(FALSE ("DTResetEncoder")) -> ()
          n870 = global write "Robot Global Data.vi" "AutoFlyw"(FALSE ("DTResetEncoder")) -> ()
        }
        frame #7 {
          n871 = global write "Robot Global Data.vi" "AutoHopperPanelPistons"(TRUE ("GyroReset")) -> ()
          n872 = global write "Robot Global Data.vi" "AutoStep"("PID on" ("AutoStep")) -> ()
          n873 = global write "Robot Global Data.vi" "AutoAngle"(0.0 ("DriveAngle")) -> ()
          n874 = global write "Robot Global Data.vi" "FwdPIDOn"(TRUE ("FwdPIDOn")) -> ()
          n875 = global write "Robot Global Data.vi" "AutoDistance"(0.0 ("DriveDistance")) -> ()
          n876 = global write "Robot Global Data.vi" "AutoGearClamp"(TRUE ("DTResetEncoder")) -> ()
          n877 = global write "Robot Global Data.vi" "AutoGyroReset"(FALSE ("GyroReset")) -> ()
          n878 = global write "Robot Global Data.vi" "AutoIntakePistons"(FALSE ("GyroReset")) -> ()
          n879 = global write "Robot Global Data.vi" "DTResetEncoder"(FALSE ("DTResetEncoder")) -> ()
          n880 = global write "Robot Global Data.vi" "AutoAngle PIDOn"(TRUE ("AnglePIDOn")) -> ()
          n881 = global write "Robot Global Data.vi" "AutoBallIntake"(TRUE ("DTResetEncoder")) -> ()
          n882 = global write "Robot Global Data.vi" "AutoConv+Upt"(FALSE ("DTResetEncoder")) -> ()
          n883 = global write "Robot Global Data.vi" "AutoFlyw"(FALSE ("DTResetEncoder")) -> ()
          n884 = Wait (ms)(milliseconds to wait=u32 300) -> ()  [unwired: 1 out]
        }
        frame #8 {
          n885 = global write "Robot Global Data.vi" "AutoHopperPanelPistons"(TRUE ("GyroReset")) -> ()
          n886 = global write "Robot Global Data.vi" "AutoIntakePistons"(FALSE ("GyroReset")) -> ()
          n887 = global write "Robot Global Data.vi" "AutoStep"("drive fwd after turn" ("AutoStep")) -> ()
          n888 = global write "Robot Global Data.vi" "AutoAngle"(0.0 ("DriveAngle")) -> ()
          n889 = global write "Robot Global Data.vi" "FwdPIDOn"(TRUE ("FwdPIDOn")) -> ()
          n890 = global write "Robot Global Data.vi" "AutoConv+Upt"(FALSE ("DTResetEncoder")) -> ()
          n891 = global write "Robot Global Data.vi" "AutoDistance"(3468.0 ("DriveDistance")) -> ()
          n892 = global write "Robot Global Data.vi" "AutoGearClamp"(TRUE ("DTResetEncoder")) -> ()
          n893 = global write "Robot Global Data.vi" "AutoBallIntake"(TRUE ("DTResetEncoder")) -> ()
          n894 = global write "Robot Global Data.vi" "AutoGyroReset"(FALSE ("GyroReset")) -> ()
          n895 = global write "Robot Global Data.vi" "DTResetEncoder"(FALSE ("DTResetEncoder")) -> ()
          n896 = global write "Robot Global Data.vi" "AutoAngle PIDOn"(TRUE ("AnglePIDOn")) -> ()
          n897 = Wait (ms)(milliseconds to wait=u32 2500) -> ()  [unwired: 1 out]
          n898 = global write "Robot Global Data.vi" "AutoFlyw"(TRUE ("DTResetEncoder")) -> ()
        }
        frame #9 {
          n899 = global write "Robot Global Data.vi" "AutoHopperPanelPistons"(TRUE ("GyroReset")) -> ()
          n900 = global write "Robot Global Data.vi" "AutoIntakePistons"(FALSE ("GyroReset")) -> ()
          n901 = global write "Robot Global Data.vi" "AutoBallIntake"(TRUE ("DTResetEncoder")) -> ()
          n902 = global write "Robot Global Data.vi" "AutoConv+Upt"(FALSE ("DTResetEncoder")) -> ()
          n903 = global write "Robot Global Data.vi" "AutoStep"("Fwd PID Off " ("AutoStep")) -> ()
          n904 = global write "Robot Global Data.vi" "AutoGearClamp"(TRUE ("DTResetEncoder")) -> ()
          n905 = global write "Robot Global Data.vi" "AutoAngle"(0.0 ("DriveAngle")) -> ()
          n906 = global write "Robot Global Data.vi" "FwdPIDOn"(FALSE ("FwdPIDOn")) -> ()
          n907 = global write "Robot Global Data.vi" "AutoDistance"(3468.0 ("DriveDistance")) -> ()
          n908 = global write "Robot Global Data.vi" "AutoGyroReset"(FALSE ("GyroReset")) -> ()
          n909 = global write "Robot Global Data.vi" "DTResetEncoder"(FALSE ("DTResetEncoder")) -> ()
          n910 = global write "Robot Global Data.vi" "AutoAngle PIDOn"(TRUE ("AnglePIDOn")) -> ()
          n911 = global write "Robot Global Data.vi" "AutoFlyw"(TRUE ("DTResetEncoder")) -> ()
        }
        frame #10 {
          n912 = global write "Robot Global Data.vi" "AutoHopperPanelPistons"(TRUE ("GyroReset")) -> ()
          n913 = global write "Robot Global Data.vi" "AutoIntakePistons"(FALSE ("GyroReset")) -> ()
          n914 = global write "Robot Global Data.vi" "AutoConv+Upt"(FALSE ("DTResetEncoder")) -> ()
          n915 = global write "Robot Global Data.vi" "AutoBallIntake"(TRUE ("DTResetEncoder")) -> ()
          n916 = global write "Robot Global Data.vi" "AutoStep"("Turn Right" ("AutoStep")) -> ()
          n917 = global write "Robot Global Data.vi" "AutoAngle"(-60.0 ("DriveAngle")) -> ()
          n918 = global write "Robot Global Data.vi" "FwdPIDOn"(FALSE ("FwdPIDOn")) -> ()
          n919 = global write "Robot Global Data.vi" "AutoDistance"(0.0 ("DriveDistance")) -> ()
          n920 = global write "Robot Global Data.vi" "AutoGearClamp"(TRUE ("DTResetEncoder")) -> ()
          n921 = global write "Robot Global Data.vi" "AutoGyroReset"(FALSE ("GyroReset")) -> ()
          n922 = global write "Robot Global Data.vi" "DTResetEncoder"(FALSE ("DTResetEncoder")) -> ()
          n923 = global write "Robot Global Data.vi" "AutoAngle PIDOn"(TRUE ("AnglePIDOn")) -> ()
          n924 = global write "Robot Global Data.vi" "AutoFlyw"(TRUE ("DTResetEncoder")) -> ()
          n925 = Wait (ms)(milliseconds to wait=u32 2000) -> ()  [unwired: 1 out]
        }
        frame #11 {
          n926 = global write "Robot Global Data.vi" "AutoHopperPanelPistons"(TRUE ("GyroReset")) -> ()
          n927 = global write "Robot Global Data.vi" "AutoIntakePistons"(FALSE ("GyroReset")) -> ()
          n928 = global write "Robot Global Data.vi" "AutoBallIntake"(TRUE ("DTResetEncoder")) -> ()
          n929 = global write "Robot Global Data.vi" "AutoConv+Upt"(TRUE ("DTResetEncoder")) -> ()
          n930 = global write "Robot Global Data.vi" "AutoStep"("PIDs Off +shoot  " ("AutoStep")) -> ()
          n931 = global write "Robot Global Data.vi" "AutoAngle"(-60.0 ("DriveAngle")) -> ()
          n932 = global write "Robot Global Data.vi" "FwdPIDOn"(FALSE ("FwdPIDOn")) -> ()
          n933 = global write "Robot Global Data.vi" "AutoDistance"(0.0 ("DriveDistance")) -> ()
          n934 = global write "Robot Global Data.vi" "AutoGearClamp"(FALSE ("DTResetEncoder")) -> ()
          n935 = global write "Robot Global Data.vi" "AutoGyroReset"(FALSE ("GyroReset")) -> ()
          n936 = global write "Robot Global Data.vi" "DTResetEncoder"(FALSE ("DTResetEncoder")) -> ()
          n937 = global write "Robot Global Data.vi" "AutoAngle PIDOn"(FALSE ("AnglePIDOn")) -> ()
          n938 = global write "Robot Global Data.vi" "AutoFlyw"(TRUE ("DTResetEncoder")) -> ()
          n939 = Wait (ms)(milliseconds to wait=u32 1000) -> ()  [unwired: 1 out]
        }
        frame #12 {
          n940 = global write "Robot Global Data.vi" "AutoHopperPanelPistons"(TRUE ("GyroReset")) -> ()
          n941 = global write "Robot Global Data.vi" "AutoIntakePistons"(FALSE ("GyroReset")) -> ()
          n942 = global write "Robot Global Data.vi" "AutoStep"("reset+stop" ("AutoStep")) -> ()
          n943 = global write "Robot Global Data.vi" "AutoAngle"(0.0 ("DriveAngle")) -> ()
          n944 = global write "Robot Global Data.vi" "FwdPIDOn"(FALSE ("FwdPIDOn")) -> ()
          n945 = global write "Robot Global Data.vi" "AutoDistance"(0.0 ("DriveDistance")) -> ()
          n946 = global write "Robot Global Data.vi" "AutoGearClamp"(FALSE ("DTResetEncoder")) -> ()
          n947 = global write "Robot Global Data.vi" "AutoGyroReset"(TRUE ("GyroReset")) -> ()
          n948 = global write "Robot Global Data.vi" "DTResetEncoder"(TRUE ("DTResetEncoder")) -> ()
          n949 = global write "Robot Global Data.vi" "AutoAngle PIDOn"(FALSE ("AnglePIDOn")) -> ()
          n950 = global write "Robot Global Data.vi" "AutoConv+Upt"(FALSE ("DTResetEncoder")) -> ()
          n951 = global write "Robot Global Data.vi" "AutoBallIntake"(FALSE ("DTResetEncoder")) -> ()
          n952 = global write "Robot Global Data.vi" "AutoFlyw"(FALSE ("DTResetEncoder")) -> ()
          n953 = Wait (ms)(milliseconds to wait=u32 500) -> ()  [unwired: 1 out]
        }
        frame #13 {
          n954 = global write "Robot Global Data.vi" "AutoHopperPanelPistons"(TRUE ("GyroReset")) -> ()
          n955 = global write "Robot Global Data.vi" "AutoIntakePistons"(FALSE ("GyroReset")) -> ()
          n956 = global write "Robot Global Data.vi" "AutoStep"("stop" ("AutoStep")) -> ()
          n957 = global write "Robot Global Data.vi" "AutoAngle"(0.0 ("DriveAngle")) -> ()
          n958 = global write "Robot Global Data.vi" "FwdPIDOn"(FALSE ("FwdPIDOn")) -> ()
          n959 = global write "Robot Global Data.vi" "AutoDistance"(0.0 ("DriveDistance")) -> ()
          n960 = global write "Robot Global Data.vi" "AutoGearClamp"(FALSE ("DTResetEncoder")) -> ()
          n961 = global write "Robot Global Data.vi" "AutoGyroReset"(FALSE ("GyroReset")) -> ()
          n962 = global write "Robot Global Data.vi" "DTResetEncoder"(FALSE ("DTResetEncoder")) -> ()
          n963 = global write "Robot Global Data.vi" "AutoAngle PIDOn"(FALSE ("AnglePIDOn")) -> ()
          n964 = global write "Robot Global Data.vi" "AutoBallIntake"(FALSE ("DTResetEncoder")) -> ()
          n965 = global write "Robot Global Data.vi" "AutoConv+Upt"(FALSE ("DTResetEncoder")) -> ()
          n966 = global write "Robot Global Data.vi" "AutoFlyw"(FALSE ("DTResetEncoder")) -> ()
          n967 = Wait (ms)(milliseconds to wait=u32 500) -> ()  [unwired: 1 out]
        }
      }
    }
    frame "No Auto", Default {
    }
    frame "Forward On Time" {
      n968 = flat-sequence {
        tunnel: [w968] -> w959
        tunnel: w959 -> [w972]
        frame #0 {
          n969 = global write "Robot Global Data.vi" "FwdPIDOn"(FALSE ("FwdPIDOn")) -> ()
          n970 = global write "Robot Global Data.vi" "AutoHopperPanelPistons"(TRUE ("DTResetEncoder")) -> ()
          n971 = global write "Robot Global Data.vi" "DTResetEncoder"(TRUE ("DTResetEncoder")) -> ()
          n972 = global write "Robot Global Data.vi" "AutoGearClamp"(TRUE ("DTResetEncoder")) -> ()
          n973 = global write "Robot Global Data.vi" "AutoAngle PIDOn"(FALSE ("AnglePIDOn")) -> ()
          n974 = global write "Robot Global Data.vi" "AutoYAxis"(0.0 ("AutoYAxis")) -> ()
          n975 = Wait (ms)(milliseconds to wait=u32 200) -> ()  [unwired: 1 out]
        }
        frame #1 {
          n976 = global write "Robot Global Data.vi" "DTResetEncoder"(FALSE ("DTResetEncoder")) -> ()
          n977 = global write "Robot Global Data.vi" "AutoGearClamp"(TRUE ("DTResetEncoder")) -> ()
          n978 = global write "Robot Global Data.vi" "AutoYAxis"(0.6 ("AutoYAxis")) -> ()
          n979 = Wait (ms)(milliseconds to wait=u32 200) -> ()  [unwired: 1 out]
          n980 = Tick Count (ms)() -> (millisecond timer value=w968:u32)
        }
        frame #2 {
          n981 = while {
            tunnel: w972 -> [w978]
            stop <- w980 stop-if-true
            n982 = Tick Count (ms)() -> (millisecond timer value=w979:u32)
            n983 = global read "Robot Global Data.vi" "DTEncoder Avg"() -> (w983:dbl)
            n984 = global write "Robot Global Data.vi" "AutoGearClamp"(TRUE ("DTResetEncoder")) -> ()
            n985 = Subtract(x=w979, y=w978) -> (x-y=w977:u32)
            n986 = Greater Or Equal?(x=w977, y=u32 4500) -> (x >= y?=w974:bool)
            n987 = Greater Or Equal?(x=w983, y=u32 4490 ("milliseconds to wait")) -> (x >= y?=w975:bool)
            n988 = case shown="False" w975 {
              frame False {
                n989 = global write "Robot Global Data.vi" "AutoYAxis"(0.6 ("AutoYAxis")) -> ()
              }
              frame True {
                n990 = global write "Robot Global Data.vi" "AutoYAxis"(0.0 ("AutoYAxis")) -> ()
              }
            }
            n991 = Or(x=w975, y=w974) -> (x .or. y?=w980:bool)
            n992 = Wait (ms)(milliseconds to wait=u32 100) -> ()  [unwired: 1 out]
          }
        }
        frame #3 {
          n993 = global write "Robot Global Data.vi" "AutoGearClamp"(TRUE ("DTResetEncoder")) -> ()
          n994 = global write "Robot Global Data.vi" "DTResetEncoder"(FALSE ("DTResetEncoder")) -> ()
          n995 = global write "Robot Global Data.vi" "AutoYAxis"(0.0 ("AutoYAxis")) -> ()
          n996 = Wait (ms)(milliseconds to wait=u32 200) -> ()  [unwired: 1 out]
        }
      }
    }
  }
